vi "House.vi"() -> ()   [LabVIEW 2011]
panel:
  in  "WindowsMediaPlayer 2":refnum<k7>(container)
  out "Boolean 54":bool
  out "Boolean 53":bool
  out "Boolean 52":bool
  in  "stop 3":bool
  out "Boolean 51":bool
  out "LivingRoom2 Temprature":i32(slide) scale=1.0..60.0
  out "Bedroom2 Temprature":i32(slide) scale=1.0..60.0
  out "MasterRoom Temprature":i32(slide) scale=1.0..60.0
  out "DiningRoom Temprature":i32(slide) scale=1.0..60.0
  out "LivingRoom Temprature":i32(slide) scale=1.0..60.0
  in  "WindowsMediaPlayer":refnum<k7>(container)
  in  "stop 2":bool
  out "Bedroom Temprature":i32(slide) scale=1.0..60.0
  out "Boolean 50":bool
  out "Boolean 49":bool
  out "Boolean 48":bool
  out "Boolean 47":bool
  out "Boolean 46":bool
  out "Boolean 45":bool
  out "Slide 25":u8(slide)
  out "Slide 27":u8(slide)
  out "Horizontal Progress Bar":u8(slide) scale=0.0..100.0
  out "Horizontal Progress Bar 2":u8(slide)
  out "Boolean 44":bool
  out "Boolean 43":bool
  out "Boolean 42":bool
  out "Boolean 41":bool
  out "Boolean 40":bool
  out "Boolean 39":bool
  out "Boolean 38":bool
  out "Slide 24":u8(slide)
  out "Slide 23":u8(slide) scale=0.0..100.0
  out "Slide 22":u8(slide) scale=0.0..100.0
  out "Slide 21":u8(slide)
  out "Slide 20":u8(slide)
  out "Slide 19":u8(slide) scale=0.0..100.0
  out "Slide 18":u8(slide)
  out "Slide 17":u8(slide) scale=0.0..100.0
  out "Slide 16":u8(slide) scale=0.0..100.0
  out "Slide 15":u8(slide)
  out "Slide 14":u8(slide) scale=0.0..100.0
  out "Slide 13":u8(slide)
  out "Slide 12":u8(slide) scale=0.0..100.0
  out "Slide 11":u8(slide)
  out "Boolean 37":bool
  out "Boolean 36":bool
  out "Boolean 35":bool
  out "Boolean 34":bool
  out "Boolean 33":bool
  out "Boolean 32":bool
  out "Boolean 31":bool
  out "Boolean 30":bool
  out "Boolean 29":bool
  out "Boolean 28":bool
  out "Boolean 27":bool
  out "Slide 10":u8(slide) scale=0.0..100.0
  out "Slide 9":u8(slide)
  out "Slide 8":u8(slide)
  out "Slide 7":u8(slide) scale=0.0..100.0
  out "Slide 6":u8(slide)
  out "Slide 5":u8(slide) scale=0.0..100.0
  out "Slide 4":u8(slide) scale=0.0..100.0
  out "Slide 3":u8(slide)
  out "Slide 2":u8(slide)
  out "Slide":u8(slide) scale=0.0..100.0
  out "Boolean 26":bool
  out "Boolean 25":bool
  out "Boolean 24":bool
  out "Boolean 23":bool
  out "Boolean 22":bool
  out "Boolean 21":bool
  out "Boolean 20":bool
  out "Boolean 19":bool
  out "Boolean 18":bool
  out "Boolean 17":bool
  out "Boolean 16":bool
  out "Boolean 15":bool
  out "Boolean 14":bool
  out "Boolean 13":bool
  out "Boolean 12":bool
  out "Boolean 11":bool
  out "Boolean 10":bool
  out "Boolean 9":bool
  out "Boolean 8":bool
  out "Boolean 7":bool
  out "Boolean 6":bool
  out "Boolean 5":bool
  out "Boolean 4":bool
  out "Boolean 3":bool
  out "Boolean 2":bool
  out "Boolean":bool
  in  "stop":bool
  # "Ground Floor"
  # "First Floor"
  # "Ground Floor"
  # "First Floor"
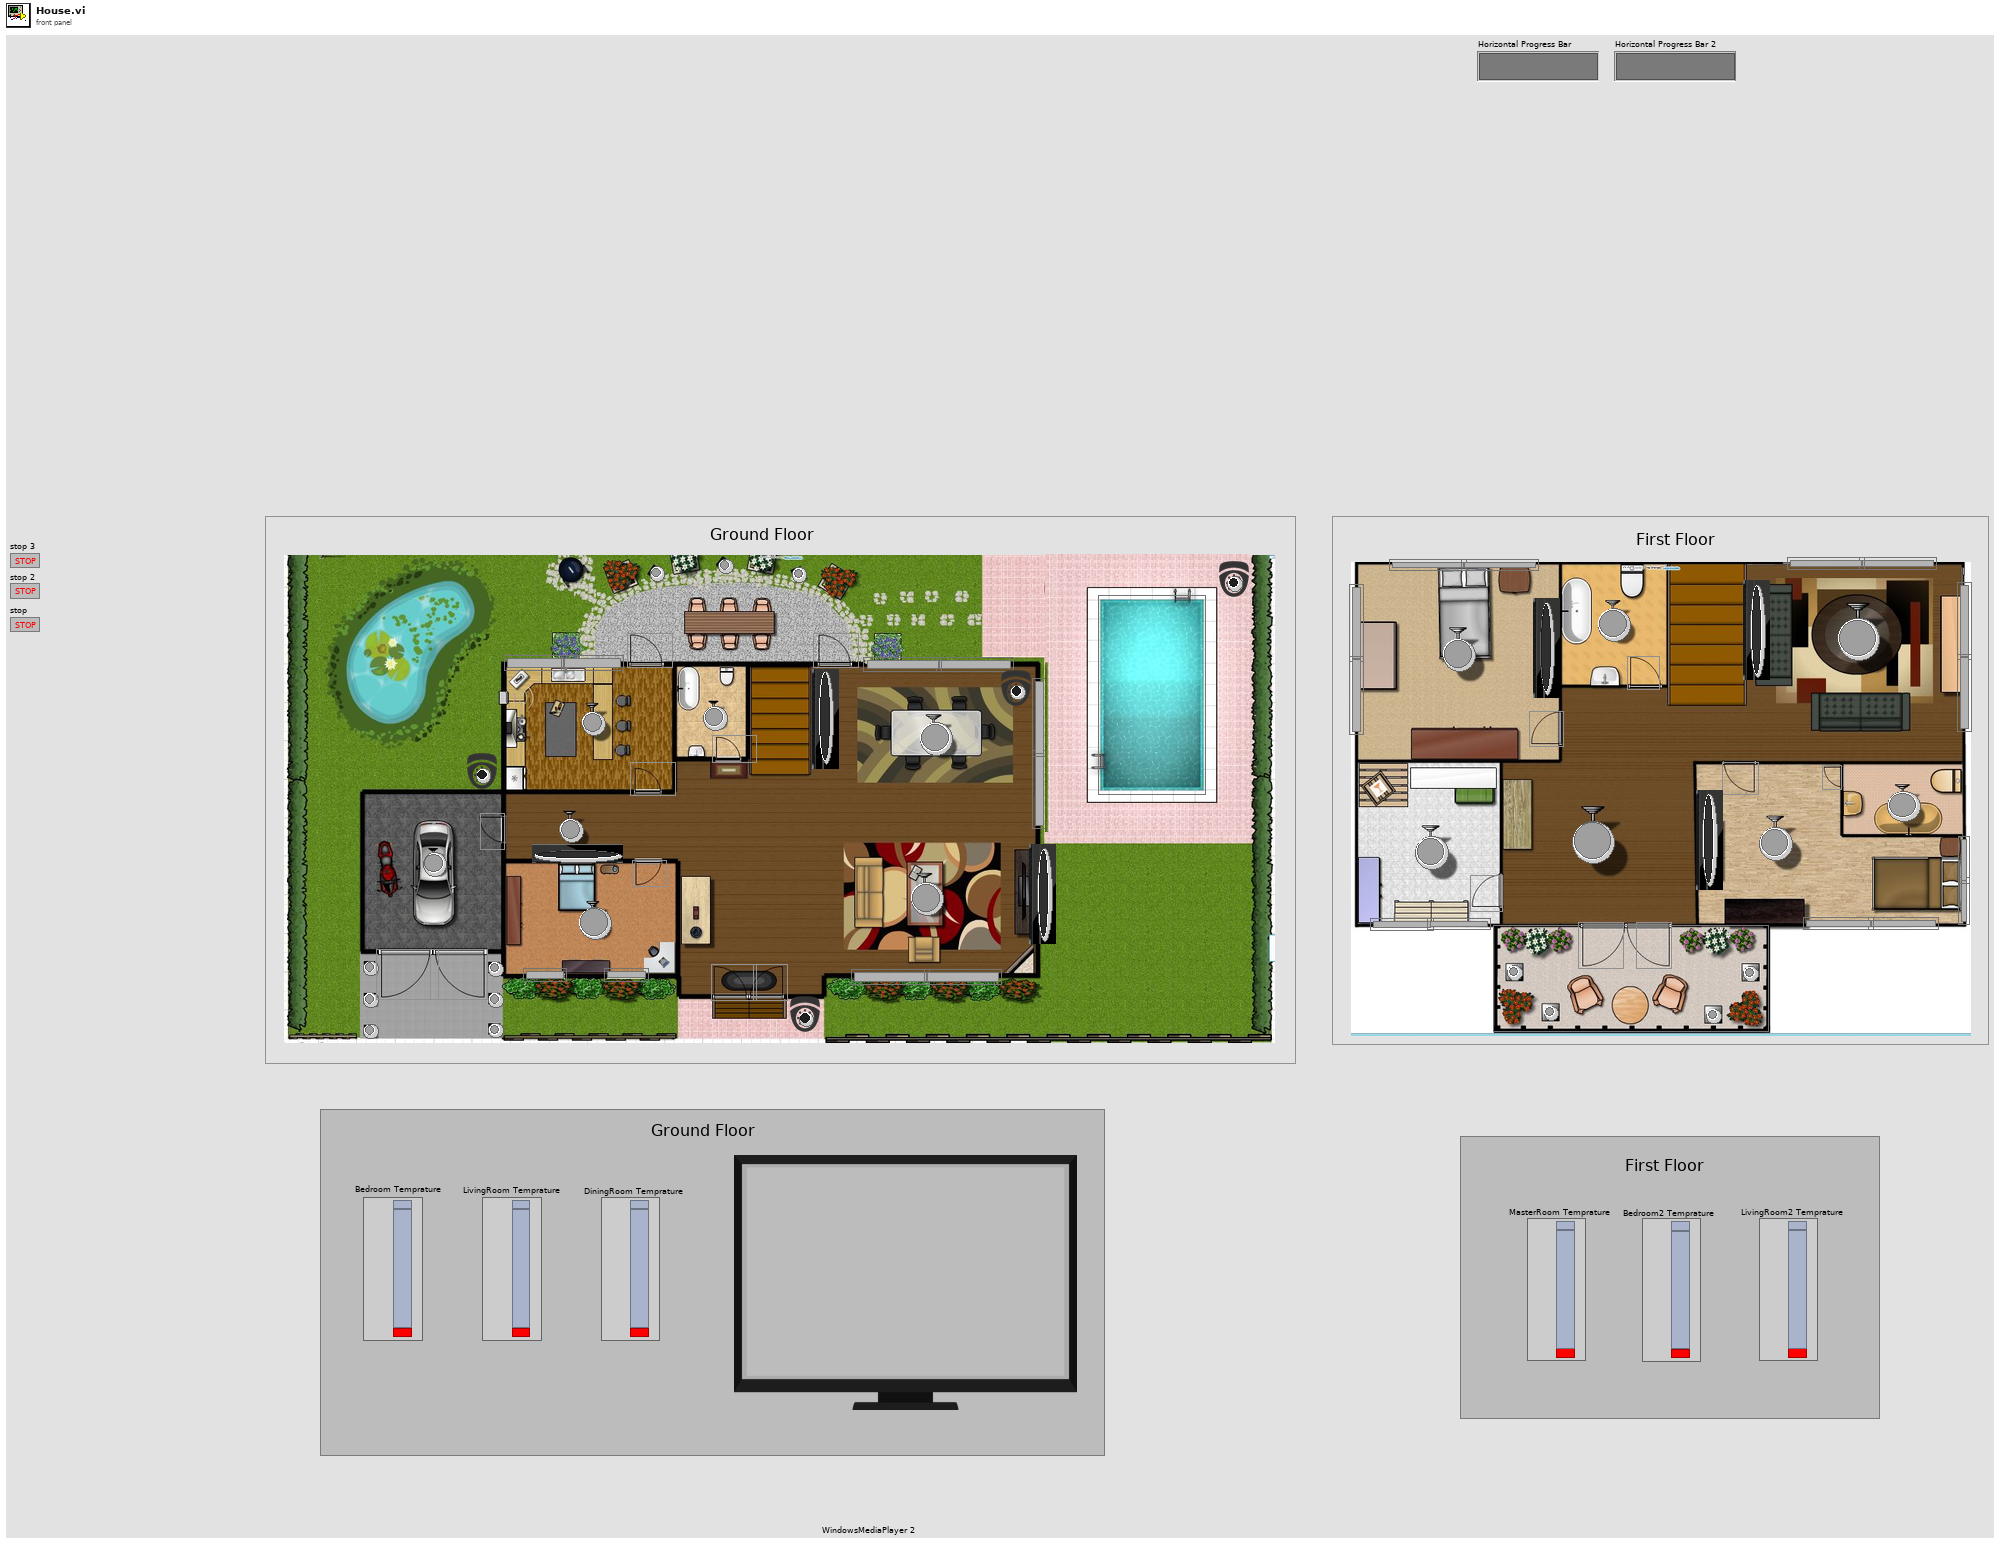
[diagram p1: front panel]
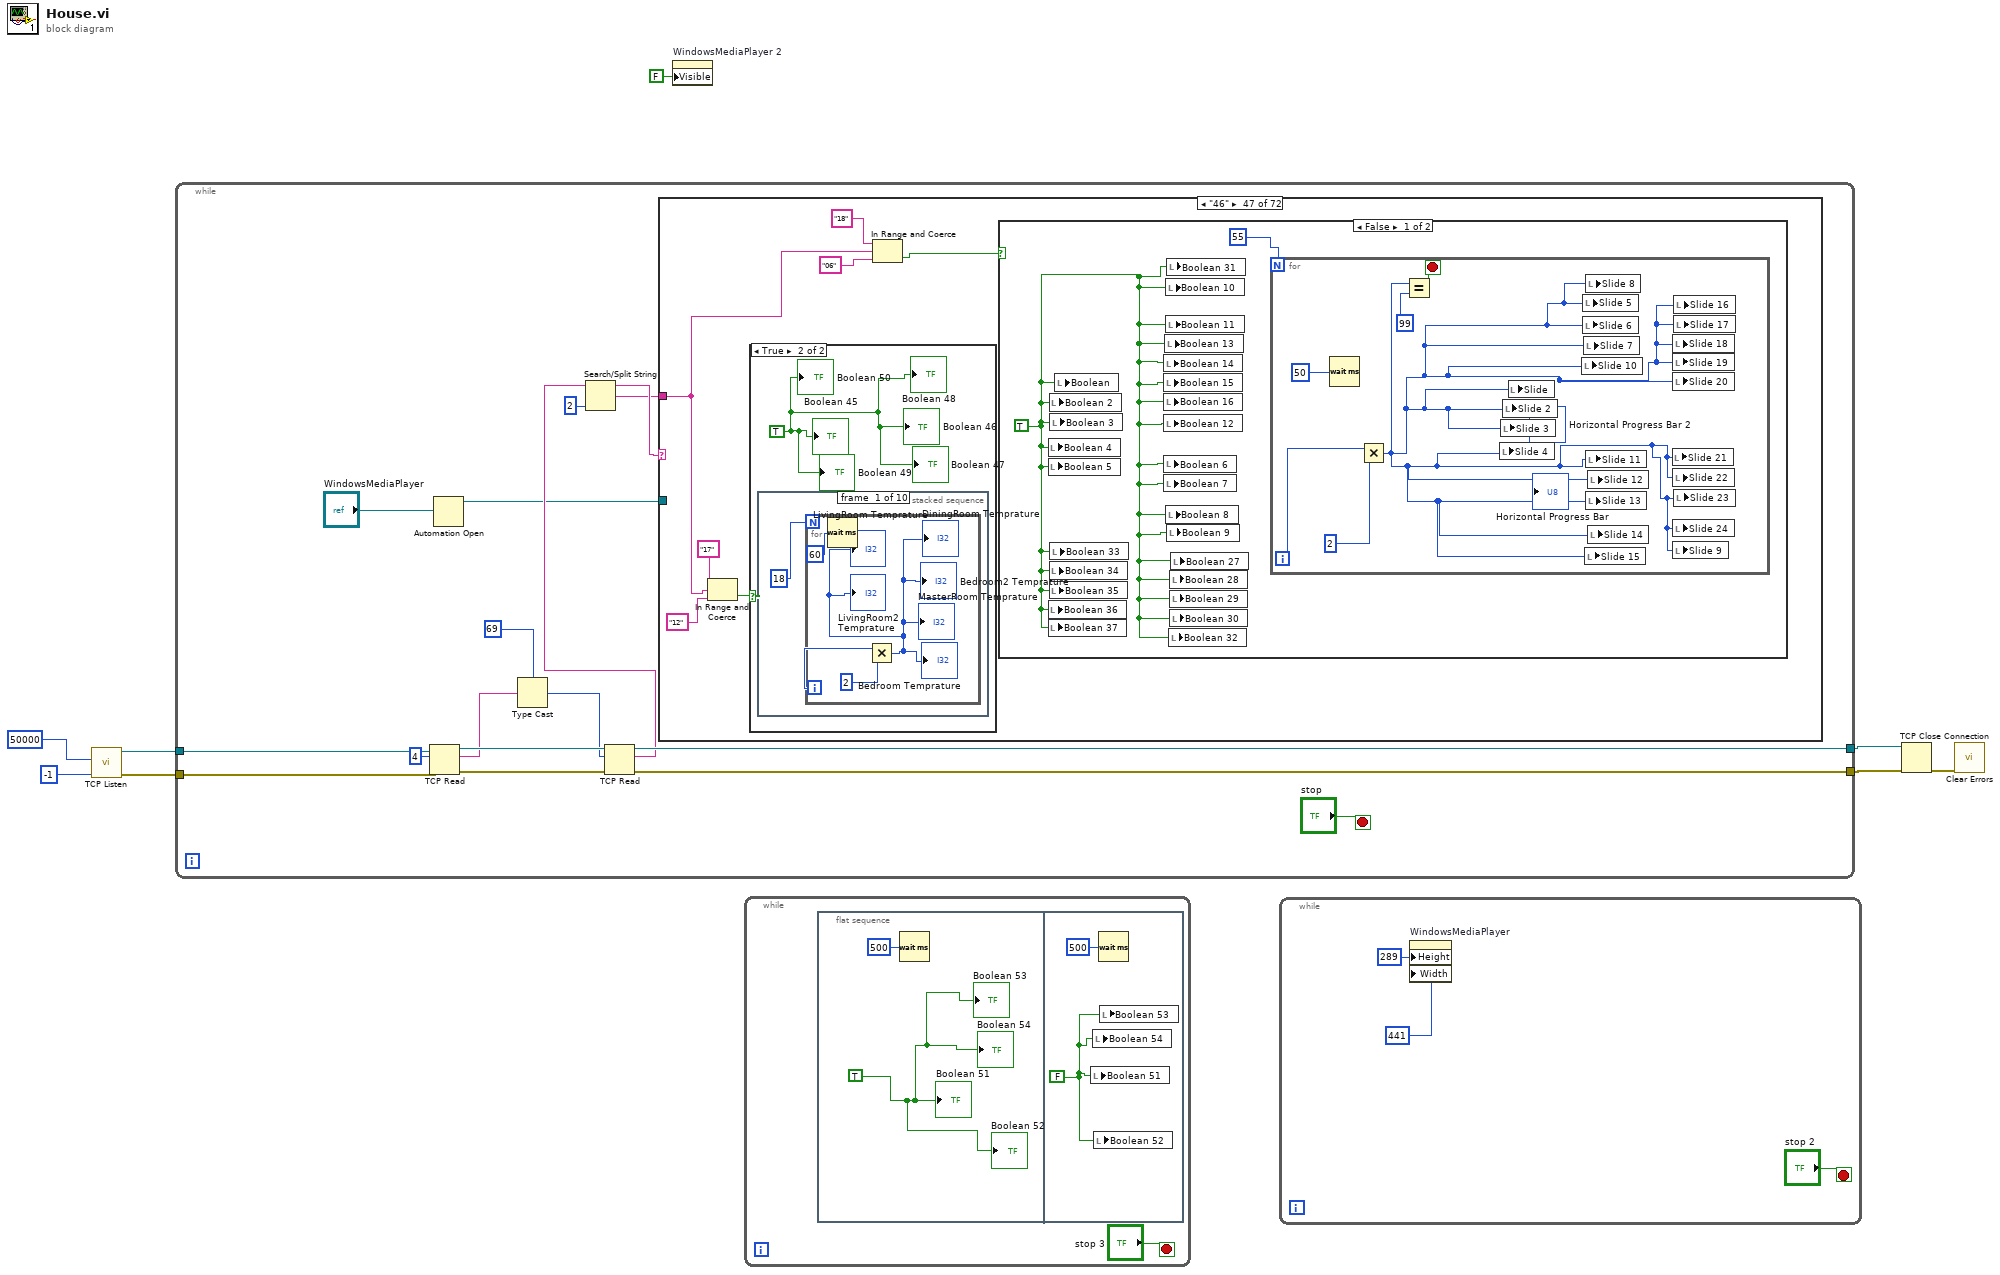
[diagram p0: block diagram]
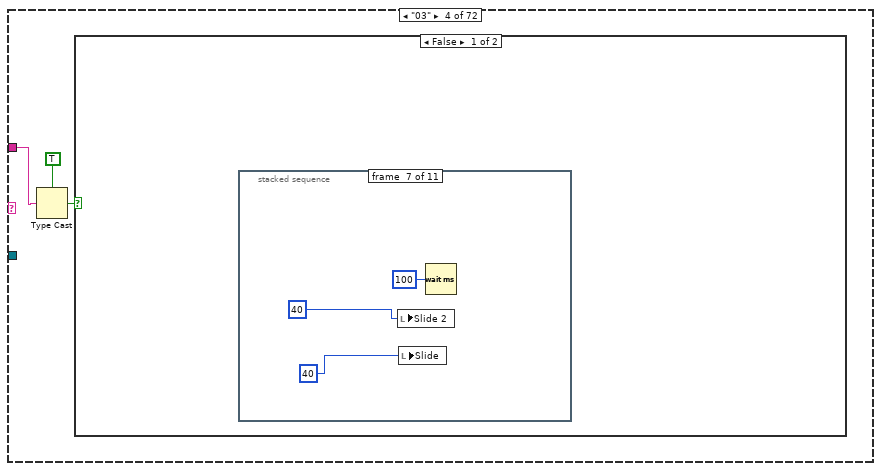
[diagram p5: hidden frame]
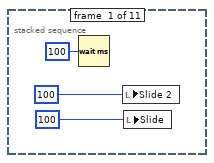
[diagram p6: hidden frame]
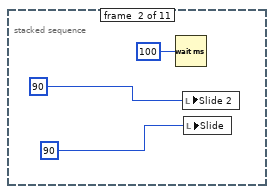
[diagram p7: hidden frame]
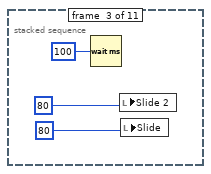
[diagram p8: hidden frame]
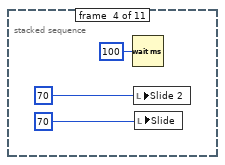
[diagram p9: hidden frame]
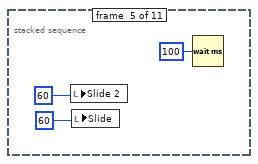
[diagram p10: hidden frame]
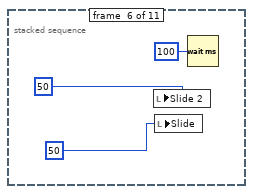
[diagram p11: hidden frame]
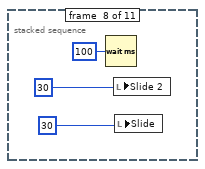
[diagram p12: hidden frame]
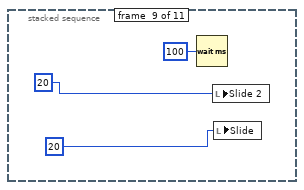
[diagram p13: hidden frame]
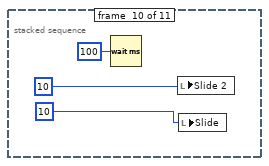
[diagram p14: hidden frame]
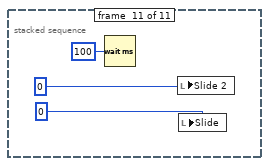
[diagram p15: hidden frame]
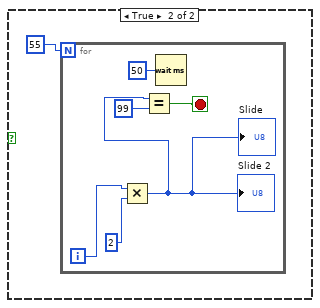
[diagram p16: hidden frame]
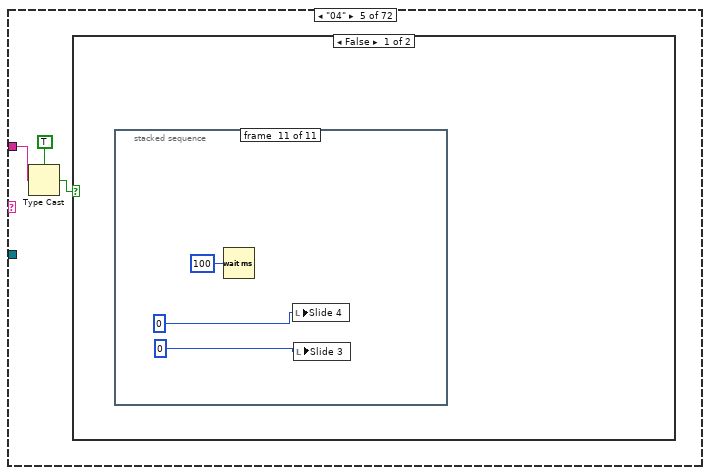
[diagram p17: hidden frame]
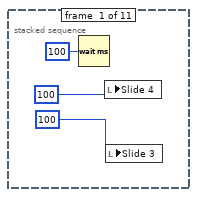
[diagram p18: hidden frame]
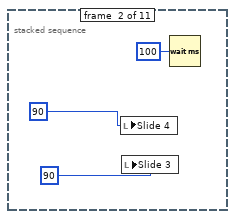
[diagram p19: hidden frame]
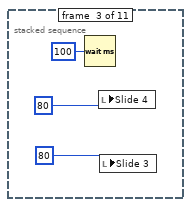
[diagram p20: hidden frame]
diagram:
  n1 = call <vilib>:"TCP Listen.vi"("timeout ms (wait forever: -1)"=-1, "port"=u16 50000) -> ("error out"=w6:errorcluster, "connection ID"=w8:refnum<k5>)  [unwired: 5 in, 3 out]
  n2 = while {
    tunnel: w8 -> [w25]
    tunnel: [w23] -> w7
    tunnel: w6 -> [w22]
    tunnel: [w9] -> w5
    stop <- "stop" stop-if-true
    n3 = TCP Read(connection ID=w25, bytes to read=4, error in (no error)=w22) -> (connection ID out=w24:refnum<k5>, data out=w19:string, error out=w21:errorcluster)  [unwired: 2 in]
    n4 = Automation Open(Automation Refnum="WindowsMediaPlayer") -> (Automation Refnum=w10:refnum<k7>)  [unwired: 3 in, 1 out]
    n5 = Type Cast(type=69, x=w19) -> (*(type *) &x=w18:i32)
    n6 = TCP Read(connection ID=w24, bytes to read=w18, error in (no error)=w21) -> (connection ID out=w23:refnum<k5>, data out=w15:string, error out=w9:errorcluster)  [unwired: 2 in]
    n7 = Search/Split String(string=w15, offset (0)=2) -> (substring before match=w13:string, match + rest of string=w12:string)  [unwired: 1 in, 1 out]
    n8 = case shown="\"46\"" w13 {
      tunnel: w12 -> [_ _ _ w27 w69 w112 w155 w199 w230 w263 w266 w269 w272 w275 w278 w281 w284 w298 w300 w303 w306 w309 w312 w315 w318 w321 w323 w355 w387 w420 w451 w483 w516 w519 w522 w525 w528 w531 w534 w537 w540 w543 w546 w549 w552 w555 w559 _ _ _ _ _ w635 w640 _ _ _ _ w654 w686 w719 w721 w723 w725 w727 w729 w731 w734 w737 w740 w743 w746]
      tunnel: w10 -> [_ _ _ _ _ _ _ _ _ _ _ _ _ _ _ _ _ _ _ _ _ _ _ _ _ _ _ _ _ _ _ _ _ _ _ _ _ _ _ _ _ _ _ _ _ _ _ w623 w626 w628 w630 w632 w638 w642 w644 w646 w648 w651 _ _ _ _ _ _ _ _ _ _ _ _ _ _]
      frame "False", Default {
      }
      frame "01" {
      }
      frame "02" {
      }
      frame "03" {
        n9 = Type Cast(type=TRUE, x=w27) -> (*(type *) &x=w28:bool)
        n10 = case shown="False" w28 {
          frame False {
            n11 = stacked-sequence {
              frame #0 {
                n12 = Wait (ms)(milliseconds to wait=u32 100) -> ()  [unwired: 1 out]
                n13 = local write "Slide 2"(u8 100 ("Horizontal Progress Bar 2")) -> ()
                n14 = local write "Slide"(u8 100 ("Horizontal Progress Bar")) -> ()
              }
              frame #1 {
                n15 = Wait (ms)(milliseconds to wait=u32 100) -> ()  [unwired: 1 out]
                n16 = local write "Slide 2"(u8 90 ("Horizontal Progress Bar 2")) -> ()
                n17 = local write "Slide"(u8 90 ("Horizontal Progress Bar")) -> ()
              }
              frame #2 {
                n18 = Wait (ms)(milliseconds to wait=u32 100) -> ()  [unwired: 1 out]
                n19 = local write "Slide 2"(u8 80 ("Horizontal Progress Bar 2")) -> ()
                n20 = local write "Slide"(u8 80 ("Horizontal Progress Bar")) -> ()
              }
              frame #3 {
                n21 = Wait (ms)(milliseconds to wait=u32 100) -> ()  [unwired: 1 out]
                n22 = local write "Slide 2"(u8 70 ("Horizontal Progress Bar 2")) -> ()
                n23 = local write "Slide"(u8 70 ("Horizontal Progress Bar")) -> ()
              }
              frame #4 {
                n24 = local write "Slide 2"(u8 60 ("Horizontal Progress Bar 2")) -> ()
                n25 = local write "Slide"(u8 60 ("Horizontal Progress Bar")) -> ()
                n26 = Wait (ms)(milliseconds to wait=u32 100) -> ()  [unwired: 1 out]
              }
              frame #5 {
                n27 = local write "Slide 2"(u8 50 ("Horizontal Progress Bar 2")) -> ()
                n28 = local write "Slide"(u8 50 ("Horizontal Progress Bar")) -> ()
                n29 = Wait (ms)(milliseconds to wait=u32 100) -> ()  [unwired: 1 out]
              }
              frame #6 {
                n30 = local write "Slide 2"(u8 40 ("Horizontal Progress Bar 2")) -> ()
                n31 = local write "Slide"(u8 40 ("Horizontal Progress Bar")) -> ()
                n32 = Wait (ms)(milliseconds to wait=u32 100) -> ()  [unwired: 1 out]
              }
              frame #7 {
                n33 = Wait (ms)(milliseconds to wait=u32 100) -> ()  [unwired: 1 out]
                n34 = local write "Slide 2"(u8 30 ("Horizontal Progress Bar 2")) -> ()
                n35 = local write "Slide"(u8 30 ("Horizontal Progress Bar")) -> ()
              }
              frame #8 {
                n36 = Wait (ms)(milliseconds to wait=u32 100) -> ()  [unwired: 1 out]
                n37 = local write "Slide 2"(u8 20 ("Horizontal Progress Bar 2")) -> ()
                n38 = local write "Slide"(u8 20 ("Horizontal Progress Bar")) -> ()
              }
              frame #9 {
                n39 = Wait (ms)(milliseconds to wait=u32 100) -> ()  [unwired: 1 out]
                n40 = local write "Slide 2"(u8 10 ("Horizontal Progress Bar 2")) -> ()
                n41 = local write "Slide"(u8 10 ("Horizontal Progress Bar")) -> ()
              }
              frame #10 {
                n42 = Wait (ms)(milliseconds to wait=u32 100) -> ()  [unwired: 1 out]
                n43 = local write "Slide 2"(u8 0 ("Horizontal Progress Bar 2")) -> ()
                n44 = local write "Slide"(u8 0 ("Horizontal Progress Bar")) -> ()
              }
            }
          }
          frame True {
            n45 = for {
              N: 55 -> [_]
              i -> [w68]
              stop <- w64 stop-if-true
              n46 = Multiply(x=w68, y=2) -> (x*y=w66:i32)
              "Slide" <- w66
              "Slide 2" <- w66
              n47 = Equal?(x=w66, y=99) -> (x = y?=w64:bool)
              n48 = Wait (ms)(milliseconds to wait=u32 50) -> ()  [unwired: 1 out]
            }
          }
        }
      }
      frame "04" {
        n49 = Type Cast(type=TRUE, x=w69) -> (*(type *) &x=w70:bool)
        n50 = case shown="False" w70 {
          frame False {
            n51 = stacked-sequence {
              frame #0 {
                n52 = Wait (ms)(milliseconds to wait=u32 100) -> ()  [unwired: 1 out]
                n53 = local write "Slide 4"(u8 100 ("Horizontal Progress Bar 2")) -> ()
                n54 = local write "Slide 3"(u8 100 ("Horizontal Progress Bar")) -> ()
              }
              frame #1 {
                n55 = local write "Slide 4"(u8 90 ("Horizontal Progress Bar 2")) -> ()
                n56 = local write "Slide 3"(u8 90 ("Horizontal Progress Bar")) -> ()
                n57 = Wait (ms)(milliseconds to wait=u32 100) -> ()  [unwired: 1 out]
              }
              frame #2 {
                n58 = Wait (ms)(milliseconds to wait=u32 100) -> ()  [unwired: 1 out]
                n59 = local write "Slide 4"(u8 80 ("Horizontal Progress Bar 2")) -> ()
                n60 = local write "Slide 3"(u8 80 ("Horizontal Progress Bar")) -> ()
              }
              frame #3 {
                n61 = local write "Slide 4"(u8 70 ("Horizontal Progress Bar 2")) -> ()
                n62 = local write "Slide 3"(u8 70 ("Horizontal Progress Bar")) -> ()
                n63 = Wait (ms)(milliseconds to wait=u32 100) -> ()  [unwired: 1 out]
              }
              frame #4 {
                n64 = local write "Slide 4"(u8 60 ("Horizontal Progress Bar 2")) -> ()
                n65 = local write "Slide 3"(u8 60 ("Horizontal Progress Bar")) -> ()
                n66 = Wait (ms)(milliseconds to wait=u32 100) -> ()  [unwired: 1 out]
              }
              frame #5 {
                n67 = Wait (ms)(milliseconds to wait=u32 100) -> ()  [unwired: 1 out]
                n68 = local write "Slide 4"(u8 50 ("Horizontal Progress Bar 2")) -> ()
                n69 = local write "Slide 3"(u8 50 ("Horizontal Progress Bar")) -> ()
              }
              frame #6 {
                n70 = local write "Slide 4"(u8 40 ("Horizontal Progress Bar 2")) -> ()
                n71 = local write "Slide 3"(u8 40 ("Horizontal Progress Bar")) -> ()
                n72 = Wait (ms)(milliseconds to wait=u32 100) -> ()  [unwired: 1 out]
              }
              frame #7 {
                n73 = Wait (ms)(milliseconds to wait=u32 100) -> ()  [unwired: 1 out]
                n74 = local write "Slide 4"(u8 30 ("Horizontal Progress Bar 2")) -> ()
                n75 = local write "Slide 3"(u8 30 ("Horizontal Progress Bar")) -> ()
              }
              frame #8 {
                n76 = Wait (ms)(milliseconds to wait=u32 100) -> ()  [unwired: 1 out]
                n77 = local write "Slide 4"(u8 20 ("Horizontal Progress Bar 2")) -> ()
                n78 = local write "Slide 3"(u8 20 ("Horizontal Progress Bar")) -> ()
              }
              frame #9 {
                n79 = Wait (ms)(milliseconds to wait=u32 100) -> ()  [unwired: 1 out]
                n80 = local write "Slide 4"(u8 10 ("Horizontal Progress Bar 2")) -> ()
                n81 = local write "Slide 3"(u8 10 ("Horizontal Progress Bar")) -> ()
              }
              frame #10 {
                n82 = Wait (ms)(milliseconds to wait=u32 100) -> ()  [unwired: 1 out]
                n83 = local write "Slide 4"(u8 0 ("Horizontal Progress Bar 2")) -> ()
                n84 = local write "Slide 3"(u8 0 ("Horizontal Progress Bar")) -> ()
              }
            }
          }
          frame True {
            n85 = for {
              N: 55 -> [_]
              i -> [w111]
              stop <- w108 stop-if-true
              n86 = Multiply(x=w111, y=2) -> (x*y=w106:i32)
              "Slide 3" <- w106
              "Slide 4" <- w106
              n87 = Equal?(x=w106, y=99) -> (x = y?=w108:bool)
              n88 = Wait (ms)(milliseconds to wait=u32 50) -> ()  [unwired: 1 out]
            }
          }
        }
      }
      frame "05" {
        n89 = Type Cast(type=TRUE, x=w112) -> (*(type *) &x=w113:bool)
        n90 = case shown="False" w113 {
          frame False {
            n91 = stacked-sequence {
              frame #0 {
                n92 = Wait (ms)(milliseconds to wait=u32 100) -> ()  [unwired: 1 out]
                n93 = local write "Slide 6"(u8 100 ("Horizontal Progress Bar 2")) -> ()
                n94 = local write "Slide 5"(u8 100 ("Horizontal Progress Bar")) -> ()
              }
              frame #1 {
                n95 = local write "Slide 6"(u8 90 ("Horizontal Progress Bar 2")) -> ()
                n96 = local write "Slide 5"(u8 90 ("Horizontal Progress Bar")) -> ()
                n97 = Wait (ms)(milliseconds to wait=u32 100) -> ()  [unwired: 1 out]
              }
              frame #2 {
                n98 = Wait (ms)(milliseconds to wait=u32 100) -> ()  [unwired: 1 out]
                n99 = local write "Slide 6"(u8 80 ("Horizontal Progress Bar 2")) -> ()
                n100 = local write "Slide 5"(u8 80 ("Horizontal Progress Bar")) -> ()
              }
              frame #3 {
                n101 = local write "Slide 6"(u8 70 ("Horizontal Progress Bar 2")) -> ()
                n102 = local write "Slide 5"(u8 70 ("Horizontal Progress Bar")) -> ()
                n103 = Wait (ms)(milliseconds to wait=u32 100) -> ()  [unwired: 1 out]
              }
              frame #4 {
                n104 = local write "Slide 6"(u8 60 ("Horizontal Progress Bar 2")) -> ()
                n105 = local write "Slide 5"(u8 60 ("Horizontal Progress Bar")) -> ()
                n106 = Wait (ms)(milliseconds to wait=u32 100) -> ()  [unwired: 1 out]
              }
              frame #5 {
                n107 = local write "Slide 6"(u8 50 ("Horizontal Progress Bar 2")) -> ()
                n108 = local write "Slide 5"(u8 50 ("Horizontal Progress Bar")) -> ()
                n109 = Wait (ms)(milliseconds to wait=u32 100) -> ()  [unwired: 1 out]
              }
              frame #6 {
                n110 = local write "Slide 6"(u8 40 ("Horizontal Progress Bar 2")) -> ()
                n111 = local write "Slide 5"(u8 40 ("Horizontal Progress Bar")) -> ()
                n112 = Wait (ms)(milliseconds to wait=u32 100) -> ()  [unwired: 1 out]
              }
              frame #7 {
                n113 = Wait (ms)(milliseconds to wait=u32 100) -> ()  [unwired: 1 out]
                n114 = local write "Slide 6"(u8 30 ("Horizontal Progress Bar 2")) -> ()
                n115 = local write "Slide 5"(u8 30 ("Horizontal Progress Bar")) -> ()
              }
              frame #8 {
                n116 = local write "Slide 6"(u8 20 ("Horizontal Progress Bar 2")) -> ()
                n117 = local write "Slide 5"(u8 20 ("Horizontal Progress Bar")) -> ()
                n118 = Wait (ms)(milliseconds to wait=u32 100) -> ()  [unwired: 1 out]
              }
              frame #9 {
                n119 = Wait (ms)(milliseconds to wait=u32 100) -> ()  [unwired: 1 out]
                n120 = local write "Slide 6"(u8 10 ("Horizontal Progress Bar 2")) -> ()
                n121 = local write "Slide 5"(u8 10 ("Horizontal Progress Bar")) -> ()
              }
              frame #10 {
                n122 = Wait (ms)(milliseconds to wait=u32 100) -> ()  [unwired: 1 out]
                n123 = local write "Slide 6"(u8 0 ("Horizontal Progress Bar 2")) -> ()
                n124 = local write "Slide 5"(u8 0 ("Horizontal Progress Bar")) -> ()
              }
            }
          }
          frame True {
            n125 = for {
              N: 55 -> [_]
              i -> [w154]
              stop <- w151 stop-if-true
              n126 = Multiply(x=w154, y=2) -> (x*y=w149:i32)
              "Slide 5" <- w149
              "Slide 6" <- w149
              n127 = Equal?(x=w149, y=99) -> (x = y?=w151:bool)
              n128 = Wait (ms)(milliseconds to wait=u32 50) -> ()  [unwired: 1 out]
            }
          }
        }
      }
      frame "06" {
        n129 = Type Cast(type=TRUE, x=w155) -> (*(type *) &x=w156:bool)
        n130 = case shown="False" w156 {
          frame False {
            n131 = stacked-sequence {
              frame #0 {
                n132 = Wait (ms)(milliseconds to wait=u32 100) -> ()  [unwired: 1 out]
                n133 = local write "Slide 8"(u8 100 ("Horizontal Progress Bar")) -> ()
                n134 = local write "Slide 7"(u8 100 ("Horizontal Progress Bar 2")) -> ()
              }
              frame #1 {
                n135 = Wait (ms)(milliseconds to wait=u32 100) -> ()  [unwired: 1 out]
                n136 = local write "Slide 8"(u8 90 ("Horizontal Progress Bar")) -> ()
                n137 = local write "Slide 7"(u8 90 ("Horizontal Progress Bar 2")) -> ()
              }
              frame #2 {
                n138 = Wait (ms)(milliseconds to wait=u32 100) -> ()  [unwired: 1 out]
                n139 = local write "Slide 8"(u8 80 ("Horizontal Progress Bar")) -> ()
                n140 = local write "Slide 7"(u8 80 ("Horizontal Progress Bar 2")) -> ()
              }
              frame #3 {
                n141 = Wait (ms)(milliseconds to wait=u32 100) -> ()  [unwired: 1 out]
                n142 = local write "Slide 8"(u8 70 ("Horizontal Progress Bar")) -> ()
                n143 = local write "Slide 7"(u8 70 ("Horizontal Progress Bar 2")) -> ()
              }
              frame #4 {
                n144 = local write "Slide 8"(u8 60 ("Horizontal Progress Bar")) -> ()
                n145 = Wait (ms)(milliseconds to wait=u32 100) -> ()  [unwired: 1 out]
                n146 = local write "Slide 7"(u8 60 ("Horizontal Progress Bar 2")) -> ()
              }
              frame #5 {
                n147 = Wait (ms)(milliseconds to wait=u32 100) -> ()  [unwired: 1 out]
                n148 = local write "Slide 8"(u8 50 ("Horizontal Progress Bar")) -> ()
                n149 = local write "Slide 7"(u8 50 ("Horizontal Progress Bar 2")) -> ()
              }
              frame #6 {
                n150 = Wait (ms)(milliseconds to wait=u32 100) -> ()  [unwired: 1 out]
                n151 = local write "Slide 8"(u8 40 ("Horizontal Progress Bar")) -> ()
                n152 = local write "Slide 7"(u8 40 ("Horizontal Progress Bar 2")) -> ()
              }
              frame #7 {
                n153 = Wait (ms)(milliseconds to wait=u32 100) -> ()  [unwired: 1 out]
                n154 = local write "Slide 8"(u8 30 ("Horizontal Progress Bar")) -> ()
                n155 = local write "Slide 7"(u8 30 ("Horizontal Progress Bar 2")) -> ()
              }
              frame #8 {
                n156 = local write "Slide 8"(u8 20 ("Horizontal Progress Bar")) -> ()
                n157 = Wait (ms)(milliseconds to wait=u32 100) -> ()  [unwired: 1 out]
                n158 = local write "Slide 7"(u8 20 ("Horizontal Progress Bar 2")) -> ()
              }
              frame #9 {
                n159 = Wait (ms)(milliseconds to wait=u32 100) -> ()  [unwired: 1 out]
                n160 = local write "Slide 8"(u8 10 ("Horizontal Progress Bar")) -> ()
                n161 = local write "Slide 7"(u8 10 ("Horizontal Progress Bar 2")) -> ()
              }
              frame #10 {
                n162 = Wait (ms)(milliseconds to wait=u32 100) -> ()  [unwired: 1 out]
                n163 = local write "Slide 8"(u8 0 ("Horizontal Progress Bar")) -> ()
                n164 = local write "Slide 7"(u8 0 ("Horizontal Progress Bar 2")) -> ()
              }
            }
          }
          frame True {
            n165 = for {
              N: 55 -> [_]
              i -> [w197]
              stop <- w194 stop-if-true
              n166 = Multiply(x=w197, y=2) -> (x*y=w192:i32)
              "Slide 7" <- w192
              "Slide 8" <- w192
              n167 = Equal?(x=w192, y=99) -> (x = y?=w194:bool)
              n168 = Wait (ms)(milliseconds to wait=u32 50) -> ()  [unwired: 1 out]
            }
          }
        }
      }
      frame "07" {
        n169 = Type Cast(type=TRUE, x=w199) -> (*(type *) &x=w198:bool)
        n170 = case shown="False" w198 {
          frame False {
            n171 = stacked-sequence {
              frame #0 {
                n172 = Wait (ms)(milliseconds to wait=u32 100) -> ()  [unwired: 1 out]
                n173 = local write "Slide 9"(u8 100 ("Horizontal Progress Bar 2")) -> ()
              }
              frame #1 {
                n174 = local write "Slide 9"(u8 90 ("Horizontal Progress Bar 2")) -> ()
                n175 = Wait (ms)(milliseconds to wait=u32 100) -> ()  [unwired: 1 out]
              }
              frame #2 {
                n176 = Wait (ms)(milliseconds to wait=u32 100) -> ()  [unwired: 1 out]
                n177 = local write "Slide 9"(u8 80 ("Horizontal Progress Bar 2")) -> ()
              }
              frame #3 {
                n178 = local write "Slide 9"(u8 70 ("Horizontal Progress Bar 2")) -> ()
                n179 = Wait (ms)(milliseconds to wait=u32 100) -> ()  [unwired: 1 out]
              }
              frame #4 {
                n180 = local write "Slide 9"(u8 60 ("Horizontal Progress Bar 2")) -> ()
                n181 = Wait (ms)(milliseconds to wait=u32 100) -> ()  [unwired: 1 out]
              }
              frame #5 {
                n182 = local write "Slide 9"(u8 50 ("Horizontal Progress Bar 2")) -> ()
                n183 = Wait (ms)(milliseconds to wait=u32 100) -> ()  [unwired: 1 out]
              }
              frame #6 {
                n184 = local write "Slide 9"(u8 40 ("Horizontal Progress Bar 2")) -> ()
                n185 = Wait (ms)(milliseconds to wait=u32 100) -> ()  [unwired: 1 out]
              }
              frame #7 {
                n186 = Wait (ms)(milliseconds to wait=u32 100) -> ()  [unwired: 1 out]
                n187 = local write "Slide 9"(u8 30 ("Horizontal Progress Bar 2")) -> ()
              }
              frame #8 {
                n188 = local write "Slide 9"(u8 20 ("Horizontal Progress Bar 2")) -> ()
                n189 = Wait (ms)(milliseconds to wait=u32 100) -> ()  [unwired: 1 out]
              }
              frame #9 {
                n190 = Wait (ms)(milliseconds to wait=u32 100) -> ()  [unwired: 1 out]
                n191 = local write "Slide 9"(u8 10 ("Horizontal Progress Bar 2")) -> ()
              }
              frame #10 {
                n192 = Wait (ms)(milliseconds to wait=u32 100) -> ()  [unwired: 1 out]
                n193 = local write "Slide 9"(u8 0 ("Horizontal Progress Bar 2")) -> ()
              }
            }
          }
          frame True {
            n194 = for {
              N: 55 -> [_]
              i -> [w229]
              stop <- w226 stop-if-true
              n195 = Multiply(x=w229, y=2) -> (x*y=w224:i32)
              "Slide 9" <- w224
              n196 = Equal?(x=w224, y=99) -> (x = y?=w226:bool)
              n197 = Wait (ms)(milliseconds to wait=u32 50) -> ()  [unwired: 1 out]
            }
          }
        }
      }
      frame "08" {
        n198 = Type Cast(type=TRUE, x=w230) -> (*(type *) &x=w232:bool)
        n199 = case shown="False" w232 {
          frame False {
            n200 = stacked-sequence {
              frame #0 {
                n201 = Wait (ms)(milliseconds to wait=u32 100) -> ()  [unwired: 1 out]
                n202 = local write "Slide 10"(u8 100 ("Horizontal Progress Bar 2")) -> ()
              }
              frame #1 {
                n203 = local write "Slide 10"(u8 90 ("Horizontal Progress Bar 2")) -> ()
                n204 = Wait (ms)(milliseconds to wait=u32 100) -> ()  [unwired: 1 out]
              }
              frame #2 {
                n205 = local write "Slide 10"(u8 80 ("Horizontal Progress Bar 2")) -> ()
                n206 = Wait (ms)(milliseconds to wait=u32 100) -> ()  [unwired: 1 out]
              }
              frame #3 {
                n207 = local write "Slide 10"(u8 70 ("Horizontal Progress Bar 2")) -> ()
                n208 = Wait (ms)(milliseconds to wait=u32 100) -> ()  [unwired: 1 out]
              }
              frame #4 {
                n209 = local write "Slide 10"(u8 60 ("Horizontal Progress Bar 2")) -> ()
                n210 = Wait (ms)(milliseconds to wait=u32 100) -> ()  [unwired: 1 out]
              }
              frame #5 {
                n211 = local write "Slide 10"(u8 50 ("Horizontal Progress Bar 2")) -> ()
                n212 = Wait (ms)(milliseconds to wait=u32 100) -> ()  [unwired: 1 out]
              }
              frame #6 {
                n213 = local write "Slide 10"(u8 40 ("Horizontal Progress Bar 2")) -> ()
                n214 = Wait (ms)(milliseconds to wait=u32 100) -> ()  [unwired: 1 out]
              }
              frame #7 {
                n215 = local write "Slide 10"(u8 30 ("Horizontal Progress Bar 2")) -> ()
                n216 = Wait (ms)(milliseconds to wait=u32 100) -> ()  [unwired: 1 out]
              }
              frame #8 {
                n217 = local write "Slide 10"(u8 20 ("Horizontal Progress Bar 2")) -> ()
                n218 = Wait (ms)(milliseconds to wait=u32 100) -> ()  [unwired: 1 out]
              }
              frame #9 {
                n219 = local write "Slide 10"(u8 10 ("Horizontal Progress Bar 2")) -> ()
                n220 = Wait (ms)(milliseconds to wait=u32 100) -> ()  [unwired: 1 out]
              }
              frame #10 {
                n221 = Wait (ms)(milliseconds to wait=u32 100) -> ()  [unwired: 1 out]
                n222 = local write "Slide 10"(u8 0 ("Horizontal Progress Bar 2")) -> ()
              }
            }
          }
          frame True {
            n223 = for {
              N: 55 -> [_]
              i -> [w261]
              stop <- w258 stop-if-true
              n224 = Multiply(x=w261, y=2) -> (x*y=w256:i32)
              "Slide 10" <- w256
              n225 = Equal?(x=w256, y=99) -> (x = y?=w258:bool)
              n226 = Wait (ms)(milliseconds to wait=u32 50) -> ()  [unwired: 1 out]
            }
          }
        }
      }
      frame "09" {
        n227 = Type Cast(type=TRUE, x=w263) -> (*(type *) &x=→"Boolean 17" →"Boolean 18":bool)
      }
      frame "10" {
        n228 = Type Cast(type=TRUE, x=w266) -> (*(type *) &x=→"Boolean 22":bool)
      }
      frame "11" {
        n229 = Type Cast(type=TRUE, x=w269) -> (*(type *) &x=→"Boolean 21":bool)
      }
      frame "12" {
        n230 = Type Cast(type=TRUE, x=w272) -> (*(type *) &x=→"Boolean 26":bool)
      }
      frame "13" {
        n231 = Type Cast(type=TRUE, x=w275) -> (*(type *) &x=→"Boolean 19":bool)
      }
      frame "14" {
        n232 = Type Cast(type=TRUE, x=w278) -> (*(type *) &x=→"Boolean 20":bool)
      }
      frame "15" {
        n233 = Type Cast(type=TRUE, x=w281) -> (*(type *) &x=→"Boolean 23":bool)
      }
      frame "16" {
        n234 = Type Cast(type=TRUE, x=w284) -> (*(type *) &x=w283:bool)
        n235 = case shown="True" w283 {
          frame False {
            n236 = local write "Boolean 24"(FALSE ("Boolean 24")) -> ()
            n237 = local write "Boolean 25"(FALSE ("Boolean 24")) -> ()
            n238 = local read "WindowsMediaPlayer 2"() -> (w286:refnum<k7>)
            n239 = property class="IWMPPlayer4"(reference=w286) -> ("controls"=w287:refnum<k7>)  [unwired: 1 in, 2 out]
            n240 = invoke class="IWMPControls" method="play"(reference=w287) -> ()  [unwired: 2 in, 3 out]
          }
          frame True {
            n241 = Automation Open(Automation Refnum="WindowsMediaPlayer 2") -> (Automation Refnum=w292:refnum<k7>)  [unwired: 3 in, 1 out]
            n242 = property class="IWMPPlayer4"(reference=w292, "URL"="E:\\spcc.mp3") -> ()  [unwired: 1 in, 2 out]
            n243 = property class="IWMPPlayer4"(reference=w292) -> ("controls"=w291:refnum<k7>)  [unwired: 1 in, 2 out]
            n244 = invoke class="IWMPControls" method="play"(reference=w291) -> ()  [unwired: 2 in, 3 out]
            "Boolean 25" <- TRUE ("Boolean 24")
            "Boolean 24" <- TRUE ("Boolean 24")
          }
        }
      }
      frame "17" {
        n245 = Type Cast(type=TRUE, x=w298) -> (*(type *) &x=→"Boolean":bool)
      }
      frame "18" {
        n246 = Type Cast(type=TRUE, x=w300) -> (*(type *) &x=→"Boolean 2":bool)
      }
      frame "19" {
        n247 = Type Cast(type=TRUE, x=w303) -> (*(type *) &x=→"Boolean 3":bool)
      }
      frame "20" {
        n248 = Type Cast(type=TRUE, x=w306) -> (*(type *) &x=→"Boolean 4":bool)
      }
      frame "21" {
        n249 = Type Cast(type=TRUE, x=w309) -> (*(type *) &x=→"Boolean 5":bool)
      }
      frame "22" {
        n250 = Type Cast(type=TRUE, x=w312) -> (*(type *) &x=→"Boolean 6":bool)
      }
      frame "23" {
        n251 = Type Cast(type=TRUE, x=w315) -> (*(type *) &x=→"Boolean 7":bool)
      }
      frame "24" {
        n252 = Type Cast(type=TRUE, x=w318) -> (*(type *) &x=→"Boolean 8" →"Boolean 10" →"Boolean 11" →"Boolean 12" →"Boolean 13" →"Boolean 14":bool)
      }
      frame "25" {
        n253 = Type Cast(type=TRUE, x=w321) -> (*(type *) &x=→"Boolean 9" →"Boolean 16" →"Boolean 15":bool)
      }
      frame "26" {
        n254 = Type Cast(type=TRUE, x=w323) -> (*(type *) &x=w325:bool)
        n255 = case shown="False" w325 {
          frame False {
            n256 = stacked-sequence {
              frame #0 {
                w326 = u8 100 ("Horizontal Progress Bar 2")
                n257 = Wait (ms)(milliseconds to wait=u32 100) -> ()  [unwired: 1 out]
                n258 = local write "Slide 13"(w326) -> ()
                n259 = local write "Slide 14"(w326) -> ()
                n260 = local write "Slide 11"(w326) -> ()
                n261 = local write "Slide 12"(w326) -> ()
              }
              frame #1 {
                w328 = u8 90 ("Horizontal Progress Bar 2")
                n262 = Wait (ms)(milliseconds to wait=u32 100) -> ()  [unwired: 1 out]
                n263 = local write "Slide 13"(w328) -> ()
                n264 = local write "Slide 14"(w328) -> ()
                n265 = local write "Slide 11"(w328) -> ()
                n266 = local write "Slide 12"(w328) -> ()
              }
              frame #2 {
                w330 = u8 80 ("Horizontal Progress Bar 2")
                n267 = Wait (ms)(milliseconds to wait=u32 100) -> ()  [unwired: 1 out]
                n268 = local write "Slide 13"(w330) -> ()
                n269 = local write "Slide 14"(w330) -> ()
                n270 = local write "Slide 11"(w330) -> ()
                n271 = local write "Slide 12"(w330) -> ()
              }
              frame #3 {
                w332 = u8 70 ("Horizontal Progress Bar 2")
                n272 = Wait (ms)(milliseconds to wait=u32 100) -> ()  [unwired: 1 out]
                n273 = local write "Slide 13"(w332) -> ()
                n274 = local write "Slide 14"(w332) -> ()
                n275 = local write "Slide 11"(w332) -> ()
                n276 = local write "Slide 12"(w332) -> ()
              }
              frame #4 {
                w334 = u8 60 ("Horizontal Progress Bar 2")
                n277 = Wait (ms)(milliseconds to wait=u32 100) -> ()  [unwired: 1 out]
                n278 = local write "Slide 13"(w334) -> ()
                n279 = local write "Slide 14"(w334) -> ()
                n280 = local write "Slide 11"(w334) -> ()
                n281 = local write "Slide 12"(w334) -> ()
              }
              frame #5 {
                w336 = u8 50 ("Horizontal Progress Bar 2")
                n282 = Wait (ms)(milliseconds to wait=u32 100) -> ()  [unwired: 1 out]
                n283 = local write "Slide 13"(w336) -> ()
                n284 = local write "Slide 14"(w336) -> ()
                n285 = local write "Slide 11"(w336) -> ()
                n286 = local write "Slide 12"(w336) -> ()
              }
              frame #6 {
                w338 = u8 40 ("Horizontal Progress Bar 2")
                n287 = Wait (ms)(milliseconds to wait=u32 100) -> ()  [unwired: 1 out]
                n288 = local write "Slide 13"(w338) -> ()
                n289 = local write "Slide 14"(w338) -> ()
                n290 = local write "Slide 11"(w338) -> ()
                n291 = local write "Slide 12"(w338) -> ()
              }
              frame #7 {
                w340 = u8 30 ("Horizontal Progress Bar 2")
                n292 = Wait (ms)(milliseconds to wait=u32 100) -> ()  [unwired: 1 out]
                n293 = local write "Slide 13"(w340) -> ()
                n294 = local write "Slide 14"(w340) -> ()
                n295 = local write "Slide 11"(w340) -> ()
                n296 = local write "Slide 12"(w340) -> ()
              }
              frame #8 {
                w342 = u8 20 ("Horizontal Progress Bar 2")
                n297 = Wait (ms)(milliseconds to wait=u32 100) -> ()  [unwired: 1 out]
                n298 = local write "Slide 13"(w342) -> ()
                n299 = local write "Slide 14"(w342) -> ()
                n300 = local write "Slide 11"(w342) -> ()
                n301 = local write "Slide 12"(w342) -> ()
              }
              frame #9 {
                w344 = u8 10 ("Horizontal Progress Bar 2")
                n302 = Wait (ms)(milliseconds to wait=u32 100) -> ()  [unwired: 1 out]
                n303 = local write "Slide 13"(w344) -> ()
                n304 = local write "Slide 14"(w344) -> ()
                n305 = local write "Slide 11"(w344) -> ()
                n306 = local write "Slide 12"(w344) -> ()
              }
              frame #10 {
                w346 = u8 0 ("Horizontal Progress Bar 2")
                n307 = Wait (ms)(milliseconds to wait=u32 100) -> ()  [unwired: 1 out]
                n308 = local write "Slide 13"(w346) -> ()
                n309 = local write "Slide 14"(w346) -> ()
                n310 = local write "Slide 11"(w346) -> ()
                n311 = local write "Slide 12"(w346) -> ()
              }
            }
          }
          frame True {
            n312 = for {
              N: 55 -> [_]
              i -> [w354]
              stop <- w351 stop-if-true
              n313 = Multiply(x=w354, y=2) -> (x*y=w349:i32)
              "Slide 11" <- w349
              "Slide 12" <- w349
              "Slide 14" <- w349
              "Slide 13" <- w349
              n314 = Equal?(x=w349, y=99) -> (x = y?=w351:bool)
              n315 = Wait (ms)(milliseconds to wait=u32 50) -> ()  [unwired: 1 out]
            }
          }
        }
      }
      frame "27" {
        n316 = Type Cast(type=TRUE, x=w355) -> (*(type *) &x=w356:bool)
        n317 = case shown="False" w356 {
          frame False {
            n318 = stacked-sequence {
              frame #0 {
                w358 = u8 100 ("Horizontal Progress Bar 2")
                n319 = Wait (ms)(milliseconds to wait=u32 100) -> ()  [unwired: 1 out]
                n320 = local write "Slide 15"(w358) -> ()
                n321 = local write "Slide 16"(w358) -> ()
              }
              frame #1 {
                w360 = u8 90 ("Horizontal Progress Bar 2")
                n322 = local write "Slide 15"(w360) -> ()
                n323 = local write "Slide 16"(w360) -> ()
                n324 = Wait (ms)(milliseconds to wait=u32 100) -> ()  [unwired: 1 out]
              }
              frame #2 {
                w362 = u8 80 ("Horizontal Progress Bar 2")
                n325 = Wait (ms)(milliseconds to wait=u32 100) -> ()  [unwired: 1 out]
                n326 = local write "Slide 15"(w362) -> ()
                n327 = local write "Slide 16"(w362) -> ()
              }
              frame #3 {
                w364 = u8 70 ("Horizontal Progress Bar 2")
                n328 = Wait (ms)(milliseconds to wait=u32 100) -> ()  [unwired: 1 out]
                n329 = local write "Slide 15"(w364) -> ()
                n330 = local write "Slide 16"(w364) -> ()
              }
              frame #4 {
                w366 = u8 60 ("Horizontal Progress Bar 2")
                n331 = local write "Slide 15"(w366) -> ()
                n332 = local write "Slide 16"(w366) -> ()
                n333 = Wait (ms)(milliseconds to wait=u32 100) -> ()  [unwired: 1 out]
              }
              frame #5 {
                w368 = u8 50 ("Horizontal Progress Bar 2")
                n334 = Wait (ms)(milliseconds to wait=u32 100) -> ()  [unwired: 1 out]
                n335 = local write "Slide 15"(w368) -> ()
                n336 = local write "Slide 16"(w368) -> ()
              }
              frame #6 {
                w370 = u8 40 ("Horizontal Progress Bar 2")
                n337 = Wait (ms)(milliseconds to wait=u32 100) -> ()  [unwired: 1 out]
                n338 = local write "Slide 15"(w370) -> ()
                n339 = local write "Slide 16"(w370) -> ()
              }
              frame #7 {
                w372 = u8 30 ("Horizontal Progress Bar 2")
                n340 = Wait (ms)(milliseconds to wait=u32 100) -> ()  [unwired: 1 out]
                n341 = local write "Slide 15"(w372) -> ()
                n342 = local write "Slide 16"(w372) -> ()
              }
              frame #8 {
                w374 = u8 20 ("Horizontal Progress Bar 2")
                n343 = Wait (ms)(milliseconds to wait=u32 100) -> ()  [unwired: 1 out]
                n344 = local write "Slide 15"(w374) -> ()
                n345 = local write "Slide 16"(w374) -> ()
              }
              frame #9 {
                w376 = u8 10 ("Horizontal Progress Bar 2")
                n346 = Wait (ms)(milliseconds to wait=u32 100) -> ()  [unwired: 1 out]
                n347 = local write "Slide 15"(w376) -> ()
                n348 = local write "Slide 16"(w376) -> ()
              }
              frame #10 {
                w378 = u8 0 ("Horizontal Progress Bar 2")
                n349 = Wait (ms)(milliseconds to wait=u32 100) -> ()  [unwired: 1 out]
                n350 = local write "Slide 15"(w378) -> ()
                n351 = local write "Slide 16"(w378) -> ()
              }
            }
          }
          frame True {
            n352 = for {
              N: 55 -> [_]
              i -> [w386]
              stop <- w383 stop-if-true
              n353 = Multiply(x=w386, y=2) -> (x*y=w381:i32)
              "Slide 15" <- w381
              "Slide 16" <- w381
              n354 = Equal?(x=w381, y=99) -> (x = y?=w383:bool)
              n355 = Wait (ms)(milliseconds to wait=u32 50) -> ()  [unwired: 1 out]
            }
          }
        }
      }
      frame "28" {
        n356 = Type Cast(type=TRUE, x=w387) -> (*(type *) &x=w388:bool)
        n357 = case shown="False" w388 {
          frame False {
            n358 = stacked-sequence {
              frame #0 {
                w390 = u8 100 ("Horizontal Progress Bar 2")
                n359 = Wait (ms)(milliseconds to wait=u32 100) -> ()  [unwired: 1 out]
                n360 = local write "Slide 18"(w390) -> ()
                n361 = local write "Slide 17"(w390) -> ()
              }
              frame #1 {
                w392 = u8 90 ("Horizontal Progress Bar 2")
                n362 = Wait (ms)(milliseconds to wait=u32 100) -> ()  [unwired: 1 out]
                n363 = local write "Slide 18"(w392) -> ()
                n364 = local write "Slide 17"(w392) -> ()
              }
              frame #2 {
                w394 = u8 80 ("Horizontal Progress Bar 2")
                n365 = Wait (ms)(milliseconds to wait=u32 100) -> ()  [unwired: 1 out]
                n366 = local write "Slide 18"(w394) -> ()
                n367 = local write "Slide 17"(w394) -> ()
              }
              frame #3 {
                w396 = u8 70 ("Horizontal Progress Bar 2")
                n368 = Wait (ms)(milliseconds to wait=u32 100) -> ()  [unwired: 1 out]
                n369 = local write "Slide 18"(w396) -> ()
                n370 = local write "Slide 17"(w396) -> ()
              }
              frame #4 {
                w398 = u8 60 ("Horizontal Progress Bar 2")
                n371 = Wait (ms)(milliseconds to wait=u32 100) -> ()  [unwired: 1 out]
                n372 = local write "Slide 18"(w398) -> ()
                n373 = local write "Slide 17"(w398) -> ()
              }
              frame #5 {
                w400 = u8 50 ("Horizontal Progress Bar 2")
                n374 = Wait (ms)(milliseconds to wait=u32 100) -> ()  [unwired: 1 out]
                n375 = local write "Slide 18"(w400) -> ()
                n376 = local write "Slide 17"(w400) -> ()
              }
              frame #6 {
                w402 = u8 40 ("Horizontal Progress Bar 2")
                n377 = Wait (ms)(milliseconds to wait=u32 100) -> ()  [unwired: 1 out]
                n378 = local write "Slide 18"(w402) -> ()
                n379 = local write "Slide 17"(w402) -> ()
              }
              frame #7 {
                w404 = u8 30 ("Horizontal Progress Bar 2")
                n380 = Wait (ms)(milliseconds to wait=u32 100) -> ()  [unwired: 1 out]
                n381 = local write "Slide 18"(w404) -> ()
                n382 = local write "Slide 17"(w404) -> ()
              }
              frame #8 {
                w406 = u8 20 ("Horizontal Progress Bar 2")
                n383 = Wait (ms)(milliseconds to wait=u32 100) -> ()  [unwired: 1 out]
                n384 = local write "Slide 18"(w406) -> ()
                n385 = local write "Slide 17"(w406) -> ()
              }
              frame #9 {
                w408 = u8 10 ("Horizontal Progress Bar 2")
                n386 = Wait (ms)(milliseconds to wait=u32 100) -> ()  [unwired: 1 out]
                n387 = local write "Slide 18"(w408) -> ()
                n388 = local write "Slide 17"(w408) -> ()
              }
              frame #10 {
                w410 = u8 0 ("Horizontal Progress Bar 2")
                n389 = Wait (ms)(milliseconds to wait=u32 100) -> ()  [unwired: 1 out]
                n390 = local write "Slide 18"(w410) -> ()
                n391 = local write "Slide 17"(w410) -> ()
              }
            }
          }
          frame True {
            n392 = for {
              N: 55 -> [_]
              i -> [w418]
              stop <- w415 stop-if-true
              n393 = Multiply(x=w418, y=2) -> (x*y=w413:i32)
              "Slide 18" <- w413
              "Slide 17" <- w413
              n394 = Equal?(x=w413, y=99) -> (x = y?=w415:bool)
              n395 = Wait (ms)(milliseconds to wait=u32 50) -> ()  [unwired: 1 out]
            }
          }
        }
      }
      frame "29" {
        n396 = Type Cast(type=TRUE, x=w420) -> (*(type *) &x=w419:bool)
        n397 = case shown="False" w419 {
          frame False {
            n398 = stacked-sequence {
              frame #0 {
                w422 = u8 100 ("Horizontal Progress Bar 2")
                n399 = Wait (ms)(milliseconds to wait=u32 100) -> ()  [unwired: 1 out]
                n400 = local write "Slide 19"(w422) -> ()
                n401 = local write "Slide 20"(w422) -> ()
              }
              frame #1 {
                w424 = u8 90 ("Horizontal Progress Bar 2")
                n402 = Wait (ms)(milliseconds to wait=u32 100) -> ()  [unwired: 1 out]
                n403 = local write "Slide 19"(w424) -> ()
                n404 = local write "Slide 20"(w424) -> ()
              }
              frame #2 {
                w426 = u8 80 ("Horizontal Progress Bar 2")
                n405 = Wait (ms)(milliseconds to wait=u32 100) -> ()  [unwired: 1 out]
                n406 = local write "Slide 19"(w426) -> ()
                n407 = local write "Slide 20"(w426) -> ()
              }
              frame #3 {
                w428 = u8 70 ("Horizontal Progress Bar 2")
                n408 = Wait (ms)(milliseconds to wait=u32 100) -> ()  [unwired: 1 out]
                n409 = local write "Slide 19"(w428) -> ()
                n410 = local write "Slide 20"(w428) -> ()
              }
              frame #4 {
                w430 = u8 60 ("Horizontal Progress Bar 2")
                n411 = Wait (ms)(milliseconds to wait=u32 100) -> ()  [unwired: 1 out]
                n412 = local write "Slide 19"(w430) -> ()
                n413 = local write "Slide 20"(w430) -> ()
              }
              frame #5 {
                w432 = u8 50 ("Horizontal Progress Bar 2")
                n414 = Wait (ms)(milliseconds to wait=u32 100) -> ()  [unwired: 1 out]
                n415 = local write "Slide 19"(w432) -> ()
                n416 = local write "Slide 20"(w432) -> ()
              }
              frame #6 {
                w434 = u8 40 ("Horizontal Progress Bar 2")
                n417 = Wait (ms)(milliseconds to wait=u32 100) -> ()  [unwired: 1 out]
                n418 = local write "Slide 19"(w434) -> ()
                n419 = local write "Slide 20"(w434) -> ()
              }
              frame #7 {
                w436 = u8 30 ("Horizontal Progress Bar 2")
                n420 = Wait (ms)(milliseconds to wait=u32 100) -> ()  [unwired: 1 out]
                n421 = local write "Slide 19"(w436) -> ()
                n422 = local write "Slide 20"(w436) -> ()
              }
              frame #8 {
                w438 = u8 20 ("Horizontal Progress Bar 2")
                n423 = local write "Slide 19"(w438) -> ()
                n424 = local write "Slide 20"(w438) -> ()
                n425 = Wait (ms)(milliseconds to wait=u32 100) -> ()  [unwired: 1 out]
              }
              frame #9 {
                w440 = u8 10 ("Horizontal Progress Bar 2")
                n426 = Wait (ms)(milliseconds to wait=u32 100) -> ()  [unwired: 1 out]
                n427 = local write "Slide 19"(w440) -> ()
                n428 = local write "Slide 20"(w440) -> ()
              }
              frame #10 {
                w442 = u8 0 ("Horizontal Progress Bar 2")
                n429 = Wait (ms)(milliseconds to wait=u32 100) -> ()  [unwired: 1 out]
                n430 = local write "Slide 19"(w442) -> ()
                n431 = local write "Slide 20"(w442) -> ()
              }
            }
          }
          frame True {
            n432 = for {
              N: 55 -> [_]
              i -> [w450]
              stop <- w447 stop-if-true
              n433 = Multiply(x=w450, y=2) -> (x*y=w445:i32)
              "Slide 19" <- w445
              "Slide 20" <- w445
              n434 = Equal?(x=w445, y=99) -> (x = y?=w447:bool)
              n435 = Wait (ms)(milliseconds to wait=u32 50) -> ()  [unwired: 1 out]
            }
          }
        }
      }
      frame "30" {
        n436 = Type Cast(type=TRUE, x=w451) -> (*(type *) &x=w452:bool)
        n437 = case shown="False" w452 {
          frame False {
            n438 = stacked-sequence {
              frame #0 {
                w454 = u8 100 ("Horizontal Progress Bar 2")
                n439 = Wait (ms)(milliseconds to wait=u32 100) -> ()  [unwired: 1 out]
                n440 = local write "Slide 21"(w454) -> ()
                n441 = local write "Slide 22"(w454) -> ()
              }
              frame #1 {
                w456 = u8 90 ("Horizontal Progress Bar 2")
                n442 = Wait (ms)(milliseconds to wait=u32 100) -> ()  [unwired: 1 out]
                n443 = local write "Slide 21"(w456) -> ()
                n444 = local write "Slide 22"(w456) -> ()
              }
              frame #2 {
                w458 = u8 80 ("Horizontal Progress Bar 2")
                n445 = Wait (ms)(milliseconds to wait=u32 100) -> ()  [unwired: 1 out]
                n446 = local write "Slide 21"(w458) -> ()
                n447 = local write "Slide 22"(w458) -> ()
              }
              frame #3 {
                w460 = u8 70 ("Horizontal Progress Bar 2")
                n448 = Wait (ms)(milliseconds to wait=u32 100) -> ()  [unwired: 1 out]
                n449 = local write "Slide 21"(w460) -> ()
                n450 = local write "Slide 22"(w460) -> ()
              }
              frame #4 {
                w462 = u8 60 ("Horizontal Progress Bar 2")
                n451 = local write "Slide 21"(w462) -> ()
                n452 = local write "Slide 22"(w462) -> ()
                n453 = Wait (ms)(milliseconds to wait=u32 100) -> ()  [unwired: 1 out]
              }
              frame #5 {
                w464 = u8 50 ("Horizontal Progress Bar 2")
                n454 = local write "Slide 21"(w464) -> ()
                n455 = Wait (ms)(milliseconds to wait=u32 100) -> ()  [unwired: 1 out]
                n456 = local write "Slide 22"(w464) -> ()
              }
              frame #6 {
                w466 = u8 40 ("Horizontal Progress Bar 2")
                n457 = Wait (ms)(milliseconds to wait=u32 100) -> ()  [unwired: 1 out]
                n458 = local write "Slide 21"(w466) -> ()
                n459 = local write "Slide 22"(w466) -> ()
              }
              frame #7 {
                w468 = u8 30 ("Horizontal Progress Bar 2")
                n460 = Wait (ms)(milliseconds to wait=u32 100) -> ()  [unwired: 1 out]
                n461 = local write "Slide 21"(w468) -> ()
                n462 = local write "Slide 22"(w468) -> ()
              }
              frame #8 {
                w470 = u8 20 ("Horizontal Progress Bar 2")
                n463 = local write "Slide 21"(w470) -> ()
                n464 = local write "Slide 22"(w470) -> ()
                n465 = Wait (ms)(milliseconds to wait=u32 100) -> ()  [unwired: 1 out]
              }
              frame #9 {
                w472 = u8 10 ("Horizontal Progress Bar 2")
                n466 = Wait (ms)(milliseconds to wait=u32 100) -> ()  [unwired: 1 out]
                n467 = local write "Slide 21"(w472) -> ()
                n468 = local write "Slide 22"(w472) -> ()
              }
              frame #10 {
                w474 = u8 0 ("Horizontal Progress Bar 2")
                n469 = Wait (ms)(milliseconds to wait=u32 100) -> ()  [unwired: 1 out]
                n470 = local write "Slide 21"(w474) -> ()
                n471 = local write "Slide 22"(w474) -> ()
              }
            }
          }
          frame True {
            n472 = for {
              N: 55 -> [_]
              i -> [w482]
              stop <- w479 stop-if-true
              n473 = Multiply(x=w482, y=2) -> (x*y=w477:i32)
              "Slide 21" <- w477
              "Slide 22" <- w477
              n474 = Equal?(x=w477, y=99) -> (x = y?=w479:bool)
              n475 = Wait (ms)(milliseconds to wait=u32 50) -> ()  [unwired: 1 out]
            }
          }
        }
      }
      frame "31" {
        n476 = Type Cast(type=TRUE, x=w483) -> (*(type *) &x=w484:bool)
        n477 = case shown="False" w484 {
          frame False {
            n478 = stacked-sequence {
              frame #0 {
                w486 = u8 100 ("Horizontal Progress Bar 2")
                n479 = Wait (ms)(milliseconds to wait=u32 100) -> ()  [unwired: 1 out]
                n480 = local write "Slide 24"(w486) -> ()
                n481 = local write "Slide 23"(w486) -> ()
              }
              frame #1 {
                w488 = u8 90 ("Horizontal Progress Bar 2")
                n482 = Wait (ms)(milliseconds to wait=u32 100) -> ()  [unwired: 1 out]
                n483 = local write "Slide 24"(w488) -> ()
                n484 = local write "Slide 23"(w488) -> ()
              }
              frame #2 {
                w490 = u8 80 ("Horizontal Progress Bar 2")
                n485 = Wait (ms)(milliseconds to wait=u32 100) -> ()  [unwired: 1 out]
                n486 = local write "Slide 24"(w490) -> ()
                n487 = local write "Slide 23"(w490) -> ()
              }
              frame #3 {
                w492 = u8 70 ("Horizontal Progress Bar 2")
                n488 = Wait (ms)(milliseconds to wait=u32 100) -> ()  [unwired: 1 out]
                n489 = local write "Slide 24"(w492) -> ()
                n490 = local write "Slide 23"(w492) -> ()
              }
              frame #4 {
                w494 = u8 60 ("Horizontal Progress Bar 2")
                n491 = Wait (ms)(milliseconds to wait=u32 100) -> ()  [unwired: 1 out]
                n492 = local write "Slide 24"(w494) -> ()
                n493 = local write "Slide 23"(w494) -> ()
              }
              frame #5 {
                w496 = u8 50 ("Horizontal Progress Bar 2")
                n494 = Wait (ms)(milliseconds to wait=u32 100) -> ()  [unwired: 1 out]
                n495 = local write "Slide 24"(w496) -> ()
                n496 = local write "Slide 23"(w496) -> ()
              }
              frame #6 {
                w498 = u8 40 ("Horizontal Progress Bar 2")
                n497 = Wait (ms)(milliseconds to wait=u32 100) -> ()  [unwired: 1 out]
                n498 = local write "Slide 24"(w498) -> ()
                n499 = local write "Slide 23"(w498) -> ()
              }
              frame #7 {
                w500 = u8 30 ("Horizontal Progress Bar 2")
                n500 = Wait (ms)(milliseconds to wait=u32 100) -> ()  [unwired: 1 out]
                n501 = local write "Slide 24"(w500) -> ()
                n502 = local write "Slide 23"(w500) -> ()
              }
              frame #8 {
                w502 = u8 20 ("Horizontal Progress Bar 2")
                n503 = Wait (ms)(milliseconds to wait=u32 100) -> ()  [unwired: 1 out]
                n504 = local write "Slide 24"(w502) -> ()
                n505 = local write "Slide 23"(w502) -> ()
              }
              frame #9 {
                w504 = u8 10 ("Horizontal Progress Bar 2")
                n506 = Wait (ms)(milliseconds to wait=u32 100) -> ()  [unwired: 1 out]
                n507 = local write "Slide 24"(w504) -> ()
                n508 = local write "Slide 23"(w504) -> ()
              }
              frame #10 {
                w506 = u8 0 ("Horizontal Progress Bar 2")
                n509 = Wait (ms)(milliseconds to wait=u32 100) -> ()  [unwired: 1 out]
                n510 = local write "Slide 24"(w506) -> ()
                n511 = local write "Slide 23"(w506) -> ()
              }
            }
          }
          frame True {
            n512 = for {
              N: 55 -> [_]
              i -> [w514]
              stop <- w511 stop-if-true
              n513 = Multiply(x=w514, y=2) -> (x*y=w509:i32)
              "Slide 24" <- w509
              "Slide 23" <- w509
              n514 = Equal?(x=w509, y=99) -> (x = y?=w511:bool)
              n515 = Wait (ms)(milliseconds to wait=u32 50) -> ()  [unwired: 1 out]
            }
          }
        }
      }
      frame "32" {
        n516 = Type Cast(type=TRUE, x=w516) -> (*(type *) &x=→"Boolean 38":bool)
      }
      frame "33" {
        n517 = Type Cast(type=TRUE, x=w519) -> (*(type *) &x=→"Boolean 39":bool)
      }
      frame "34" {
        n518 = Type Cast(type=TRUE, x=w522) -> (*(type *) &x=→"Boolean 43":bool)
      }
      frame "35" {
        n519 = Type Cast(type=TRUE, x=w525) -> (*(type *) &x=→"Boolean 40":bool)
      }
      frame "36" {
        n520 = Type Cast(type=TRUE, x=w528) -> (*(type *) &x=→"Boolean 44":bool)
      }
      frame "37" {
        n521 = Type Cast(type=TRUE, x=w531) -> (*(type *) &x=→"Boolean 41" →"Boolean 42":bool)
      }
      frame "38" {
        n522 = Type Cast(type=TRUE, x=w534) -> (*(type *) &x=→"Boolean 27":bool)
      }
      frame "39" {
        n523 = Type Cast(type=TRUE, x=w537) -> (*(type *) &x=→"Boolean 28":bool)
      }
      frame "40" {
        n524 = Type Cast(type=TRUE, x=w540) -> (*(type *) &x=→"Boolean 29":bool)
      }
      frame "41" {
        n525 = Type Cast(type=TRUE, x=w543) -> (*(type *) &x=→"Boolean 30":bool)
      }
      frame "42" {
        n526 = Type Cast(type=TRUE, x=w546) -> (*(type *) &x=→"Boolean 31":bool)
      }
      frame "43" {
        n527 = Type Cast(type=TRUE, x=w549) -> (*(type *) &x=→"Boolean 32":bool)
      }
      frame "44" {
        n528 = Type Cast(type=TRUE, x=w552) -> (*(type *) &x=→"Boolean 33":bool)
      }
      frame "45" {
        n529 = Type Cast(type=TRUE, x=w555) -> (*(type *) &x=→"Boolean 34" →"Boolean 35" →"Boolean 36" →"Boolean 37":bool)
      }
      frame "46" {
        n530 = In Range and Coerce(upper limit="17", x=w559, lower limit="12") -> (In Range?=w557:bool)  [unwired: 1 out]
        n531 = case shown="True" w557 {
          frame False {
            w564 = 20 ("Thermometer")
            w565 = FALSE
            n532 = local write "Boolean 46"(w565) -> ()
            n533 = local write "Boolean 49"(w565) -> ()
            n534 = local write "Boolean 50"(w565) -> ()
            n535 = local write "Boolean 45"(w565) -> ()
            n536 = local write "MasterRoom Temprature"(w564) -> ()
            n537 = local write "LivingRoom2 Temprature"(w564) -> ()
            n538 = local write "LivingRoom Temprature"(w564) -> ()
            n539 = local write "DiningRoom Temprature"(w564) -> ()
            n540 = local write "Bedroom2 Temprature"(w564) -> ()
            n541 = local write "Bedroom Temprature"(w564) -> ()
            n542 = local write "Boolean 47"(w565) -> ()
            n543 = local write "Boolean 48"(w565) -> ()
          }
          frame True {
            w566 = TRUE
            n544 = stacked-sequence {
              frame #0 {
                n545 = for {
                  N: 18 -> [_]
                  i -> [w570]
                  n546 = Wait (ms)(milliseconds to wait=u32 60) -> ()  [unwired: 1 out]
                  n547 = Multiply(x=w570, y=2) -> (x*y=→"Bedroom Temprature" →"MasterRoom Temprature" →"DiningRoom Temprature" →"Bedroom2 Temprature" →"LivingRoom2 Temprature" →"LivingRoom Temprature":i32)
                }
              }
              frame #1 {
                w573 = 35 ("Thermometer")
                n548 = local write "MasterRoom Temprature"(w573) -> ()
                n549 = local write "LivingRoom2 Temprature"(w573) -> ()
                n550 = local write "LivingRoom Temprature"(w573) -> ()
                n551 = local write "DiningRoom Temprature"(w573) -> ()
                n552 = local write "Bedroom2 Temprature"(w573) -> ()
                n553 = local write "Bedroom Temprature"(w573) -> ()
                n554 = Wait (ms)(milliseconds to wait=u32 1000) -> ()  [unwired: 1 out]
              }
              frame #2 {
                w575 = 34 ("Thermometer")
                n555 = local write "MasterRoom Temprature"(w575) -> ()
                n556 = local write "LivingRoom2 Temprature"(w575) -> ()
                n557 = local write "LivingRoom Temprature"(w575) -> ()
                n558 = local write "DiningRoom Temprature"(w575) -> ()
                n559 = local write "Bedroom2 Temprature"(w575) -> ()
                n560 = local write "Bedroom Temprature"(w575) -> ()
                n561 = Wait (ms)(milliseconds to wait=u32 1000) -> ()  [unwired: 1 out]
              }
              frame #3 {
                w577 = 32 ("Thermometer")
                n562 = local write "MasterRoom Temprature"(w577) -> ()
                n563 = local write "LivingRoom2 Temprature"(w577) -> ()
                n564 = local write "LivingRoom Temprature"(w577) -> ()
                n565 = local write "DiningRoom Temprature"(w577) -> ()
                n566 = local write "Bedroom2 Temprature"(w577) -> ()
                n567 = local write "Bedroom Temprature"(w577) -> ()
                n568 = Wait (ms)(milliseconds to wait=u32 1000) -> ()  [unwired: 1 out]
              }
              frame #4 {
                w579 = 30 ("Thermometer")
                n569 = local write "MasterRoom Temprature"(w579) -> ()
                n570 = local write "LivingRoom2 Temprature"(w579) -> ()
                n571 = local write "LivingRoom Temprature"(w579) -> ()
                n572 = local write "DiningRoom Temprature"(w579) -> ()
                n573 = local write "Bedroom2 Temprature"(w579) -> ()
                n574 = local write "Bedroom Temprature"(w579) -> ()
                n575 = Wait (ms)(milliseconds to wait=u32 1000) -> ()  [unwired: 1 out]
              }
              frame #5 {
                w581 = 28 ("Thermometer")
                n576 = local write "MasterRoom Temprature"(w581) -> ()
                n577 = local write "LivingRoom2 Temprature"(w581) -> ()
                n578 = local write "LivingRoom Temprature"(w581) -> ()
                n579 = local write "DiningRoom Temprature"(w581) -> ()
                n580 = local write "Bedroom2 Temprature"(w581) -> ()
                n581 = local write "Bedroom Temprature"(w581) -> ()
                n582 = Wait (ms)(milliseconds to wait=u32 1000) -> ()  [unwired: 1 out]
              }
              frame #6 {
                w583 = 26 ("Thermometer")
                n583 = local write "MasterRoom Temprature"(w583) -> ()
                n584 = local write "LivingRoom2 Temprature"(w583) -> ()
                n585 = local write "LivingRoom Temprature"(w583) -> ()
                n586 = local write "DiningRoom Temprature"(w583) -> ()
                n587 = local write "Bedroom2 Temprature"(w583) -> ()
                n588 = local write "Bedroom Temprature"(w583) -> ()
                n589 = Wait (ms)(milliseconds to wait=u32 1000) -> ()  [unwired: 1 out]
              }
              frame #7 {
                w585 = 24 ("Thermometer")
                n590 = local write "MasterRoom Temprature"(w585) -> ()
                n591 = local write "LivingRoom2 Temprature"(w585) -> ()
                n592 = local write "LivingRoom Temprature"(w585) -> ()
                n593 = local write "DiningRoom Temprature"(w585) -> ()
                n594 = local write "Bedroom2 Temprature"(w585) -> ()
                n595 = local write "Bedroom Temprature"(w585) -> ()
                n596 = Wait (ms)(milliseconds to wait=u32 1000) -> ()  [unwired: 1 out]
              }
              frame #8 {
                w587 = 22 ("Thermometer")
                n597 = local write "MasterRoom Temprature"(w587) -> ()
                n598 = local write "LivingRoom2 Temprature"(w587) -> ()
                n599 = local write "LivingRoom Temprature"(w587) -> ()
                n600 = local write "DiningRoom Temprature"(w587) -> ()
                n601 = local write "Bedroom2 Temprature"(w587) -> ()
                n602 = local write "Bedroom Temprature"(w587) -> ()
                n603 = Wait (ms)(milliseconds to wait=u32 1000) -> ()  [unwired: 1 out]
              }
              frame #9 {
                w588 = 20 ("Thermometer")
                n604 = local write "MasterRoom Temprature"(w588) -> ()
                n605 = local write "LivingRoom2 Temprature"(w588) -> ()
                n606 = local write "LivingRoom Temprature"(w588) -> ()
                n607 = local write "DiningRoom Temprature"(w588) -> ()
                n608 = local write "Bedroom2 Temprature"(w588) -> ()
                n609 = local write "Bedroom Temprature"(w588) -> ()
              }
            }
            "Boolean 47" <- w566
            "Boolean 46" <- w566
            "Boolean 48" <- w566
            "Boolean 50" <- w566
            "Boolean 49" <- w566
            "Boolean 45" <- w566
          }
        }
        n610 = In Range and Coerce(upper limit="18", x=w559, lower limit="06") -> (In Range?=w558:bool)  [unwired: 1 out]
        n611 = case shown="False" w558 {
          frame False {
            w589 = TRUE
            n612 = local write "Boolean 4"(w589) -> ()
            n613 = local write "Boolean 5"(w589) -> ()
            n614 = local write "Boolean 36"(w589) -> ()
            n615 = local write "Boolean 37"(w589) -> ()
            n616 = local write "Boolean 2"(w589) -> ()
            n617 = local write "Boolean 34"(w589) -> ()
            n618 = local write "Boolean 35"(w589) -> ()
            n619 = local write "Boolean 3"(w589) -> ()
            n620 = local write "Boolean 33"(w589) -> ()
            n621 = local write "Boolean"(w589) -> ()
            n622 = local write "Boolean 14"(w589) -> ()
            n623 = local write "Boolean 15"(w589) -> ()
            n624 = local write "Boolean 16"(w589) -> ()
            n625 = local write "Boolean 12"(w589) -> ()
            n626 = local write "Boolean 6"(w589) -> ()
            n627 = local write "Boolean 7"(w589) -> ()
            n628 = local write "Boolean 13"(w589) -> ()
            n629 = local write "Boolean 10"(w589) -> ()
            n630 = local write "Boolean 11"(w589) -> ()
            n631 = local write "Boolean 8"(w589) -> ()
            n632 = local write "Boolean 31"(w589) -> ()
            n633 = local write "Boolean 9"(w589) -> ()
            n634 = local write "Boolean 32"(w589) -> ()
            n635 = local write "Boolean 28"(w589) -> ()
            n636 = local write "Boolean 29"(w589) -> ()
            n637 = local write "Boolean 30"(w589) -> ()
            n638 = local write "Boolean 27"(w589) -> ()
            n639 = for {
              N: 55 -> [_]
              i -> [w595]
              stop <- w592 stop-if-true
              n640 = Wait (ms)(milliseconds to wait=u32 50) -> ()  [unwired: 1 out]
              n641 = Multiply(x=w595, y=2) -> (x*y=w591:i32)
              n642 = Equal?(x=w591, y=99) -> (x = y?=w592:bool)
              n643 = local write "Slide 4"(w591) -> ()
              n644 = local write "Slide 3"(w591) -> ()
              n645 = local write "Slide 2"(w591) -> ()
              n646 = local write "Slide"(w591) -> ()
              n647 = local write "Slide 10"(w591) -> ()
              n648 = local write "Slide 5"(w591) -> ()
              n649 = local write "Slide 6"(w591) -> ()
              n650 = local write "Slide 7"(w591) -> ()
              n651 = local write "Slide 15"(w591) -> ()
              n652 = local write "Slide 8"(w591) -> ()
              n653 = local write "Slide 11"(w591) -> ()
              n654 = local write "Slide 13"(w591) -> ()
              n655 = local write "Slide 12"(w591) -> ()
              n656 = local write "Slide 14"(w591) -> ()
              n657 = local write "Slide 21"(w591) -> ()
              n658 = local write "Slide 18"(w591) -> ()
              n659 = local write "Slide 19"(w591) -> ()
              n660 = local write "Slide 20"(w591) -> ()
              n661 = local write "Slide 22"(w591) -> ()
              n662 = local write "Slide 24"(w591) -> ()
              n663 = local write "Slide 9"(w591) -> ()
              n664 = local write "Slide 16"(w591) -> ()
              n665 = local write "Slide 17"(w591) -> ()
              n666 = local write "Slide 23"(w591) -> ()
            }
          }
          frame True {
            w597 = FALSE
            n667 = stacked-sequence {
              frame #0 {
                w598 = u8 100 ("Horizontal Progress Bar 2")
                n668 = Wait (ms)(milliseconds to wait=u32 100) -> ()  [unwired: 1 out]
                n669 = local write "Slide 4"(w598) -> ()
                n670 = local write "Slide 3"(w598) -> ()
                n671 = local write "Slide 2"(w598) -> ()
                n672 = local write "Slide"(w598) -> ()
                n673 = local write "Slide 10"(w598) -> ()
                n674 = local write "Slide 5"(w598) -> ()
                n675 = local write "Slide 6"(w598) -> ()
                n676 = local write "Slide 7"(w598) -> ()
                n677 = local write "Slide 15"(w598) -> ()
                n678 = local write "Slide 8"(w598) -> ()
                n679 = local write "Slide 11"(w598) -> ()
                n680 = local write "Slide 13"(w598) -> ()
                n681 = local write "Slide 12"(w598) -> ()
                n682 = local write "Slide 14"(w598) -> ()
                n683 = local write "Slide 21"(w598) -> ()
                n684 = local write "Slide 18"(w598) -> ()
                n685 = local write "Slide 19"(w598) -> ()
                n686 = local write "Slide 20"(w598) -> ()
                n687 = local write "Slide 22"(w598) -> ()
                n688 = local write "Slide 24"(w598) -> ()
                n689 = local write "Slide 16"(w598) -> ()
                n690 = local write "Slide 17"(w598) -> ()
                n691 = local write "Slide 23"(w598) -> ()
                n692 = local write "Slide 9"(w598) -> ()
              }
              frame #1 {
                w600 = u8 90 ("Horizontal Progress Bar 2")
                n693 = Wait (ms)(milliseconds to wait=u32 100) -> ()  [unwired: 1 out]
                n694 = local write "Slide 4"(w600) -> ()
                n695 = local write "Slide 3"(w600) -> ()
                n696 = local write "Slide 2"(w600) -> ()
                n697 = local write "Slide"(w600) -> ()
                n698 = local write "Slide 10"(w600) -> ()
                n699 = local write "Slide 5"(w600) -> ()
                n700 = local write "Slide 6"(w600) -> ()
                n701 = local write "Slide 7"(w600) -> ()
                n702 = local write "Slide 15"(w600) -> ()
                n703 = local write "Slide 8"(w600) -> ()
                n704 = local write "Slide 11"(w600) -> ()
                n705 = local write "Slide 13"(w600) -> ()
                n706 = local write "Slide 12"(w600) -> ()
                n707 = local write "Slide 14"(w600) -> ()
                n708 = local write "Slide 21"(w600) -> ()
                n709 = local write "Slide 18"(w600) -> ()
                n710 = local write "Slide 19"(w600) -> ()
                n711 = local write "Slide 20"(w600) -> ()
                n712 = local write "Slide 22"(w600) -> ()
                n713 = local write "Slide 24"(w600) -> ()
                n714 = local write "Slide 16"(w600) -> ()
                n715 = local write "Slide 17"(w600) -> ()
                n716 = local write "Slide 23"(w600) -> ()
                n717 = local write "Slide 9"(w600) -> ()
              }
              frame #2 {
                w602 = u8 80 ("Horizontal Progress Bar 2")
                n718 = Wait (ms)(milliseconds to wait=u32 100) -> ()  [unwired: 1 out]
                n719 = local write "Slide 4"(w602) -> ()
                n720 = local write "Slide 3"(w602) -> ()
                n721 = local write "Slide 2"(w602) -> ()
                n722 = local write "Slide"(w602) -> ()
                n723 = local write "Slide 10"(w602) -> ()
                n724 = local write "Slide 5"(w602) -> ()
                n725 = local write "Slide 6"(w602) -> ()
                n726 = local write "Slide 7"(w602) -> ()
                n727 = local write "Slide 15"(w602) -> ()
                n728 = local write "Slide 8"(w602) -> ()
                n729 = local write "Slide 11"(w602) -> ()
                n730 = local write "Slide 13"(w602) -> ()
                n731 = local write "Slide 12"(w602) -> ()
                n732 = local write "Slide 14"(w602) -> ()
                n733 = local write "Slide 21"(w602) -> ()
                n734 = local write "Slide 18"(w602) -> ()
                n735 = local write "Slide 19"(w602) -> ()
                n736 = local write "Slide 20"(w602) -> ()
                n737 = local write "Slide 22"(w602) -> ()
                n738 = local write "Slide 24"(w602) -> ()
                n739 = local write "Slide 16"(w602) -> ()
                n740 = local write "Slide 17"(w602) -> ()
                n741 = local write "Slide 23"(w602) -> ()
                n742 = local write "Slide 9"(w602) -> ()
              }
              frame #3 {
                w604 = u8 70 ("Horizontal Progress Bar 2")
                n743 = Wait (ms)(milliseconds to wait=u32 100) -> ()  [unwired: 1 out]
                n744 = local write "Slide 4"(w604) -> ()
                n745 = local write "Slide 3"(w604) -> ()
                n746 = local write "Slide 2"(w604) -> ()
                n747 = local write "Slide"(w604) -> ()
                n748 = local write "Slide 10"(w604) -> ()
                n749 = local write "Slide 5"(w604) -> ()
                n750 = local write "Slide 6"(w604) -> ()
                n751 = local write "Slide 7"(w604) -> ()
                n752 = local write "Slide 15"(w604) -> ()
                n753 = local write "Slide 8"(w604) -> ()
                n754 = local write "Slide 11"(w604) -> ()
                n755 = local write "Slide 13"(w604) -> ()
                n756 = local write "Slide 12"(w604) -> ()
                n757 = local write "Slide 14"(w604) -> ()
                n758 = local write "Slide 21"(w604) -> ()
                n759 = local write "Slide 18"(w604) -> ()
                n760 = local write "Slide 19"(w604) -> ()
                n761 = local write "Slide 20"(w604) -> ()
                n762 = local write "Slide 22"(w604) -> ()
                n763 = local write "Slide 24"(w604) -> ()
                n764 = local write "Slide 16"(w604) -> ()
                n765 = local write "Slide 17"(w604) -> ()
                n766 = local write "Slide 23"(w604) -> ()
                n767 = local write "Slide 9"(w604) -> ()
              }
              frame #4 {
                w606 = u8 60 ("Horizontal Progress Bar 2")
                n768 = Wait (ms)(milliseconds to wait=u32 100) -> ()  [unwired: 1 out]
                n769 = local write "Slide 4"(w606) -> ()
                n770 = local write "Slide 3"(w606) -> ()
                n771 = local write "Slide 2"(w606) -> ()
                n772 = local write "Slide"(w606) -> ()
                n773 = local write "Slide 10"(w606) -> ()
                n774 = local write "Slide 5"(w606) -> ()
                n775 = local write "Slide 6"(w606) -> ()
                n776 = local write "Slide 7"(w606) -> ()
                n777 = local write "Slide 15"(w606) -> ()
                n778 = local write "Slide 8"(w606) -> ()
                n779 = local write "Slide 11"(w606) -> ()
                n780 = local write "Slide 13"(w606) -> ()
                n781 = local write "Slide 12"(w606) -> ()
                n782 = local write "Slide 14"(w606) -> ()
                n783 = local write "Slide 21"(w606) -> ()
                n784 = local write "Slide 18"(w606) -> ()
                n785 = local write "Slide 19"(w606) -> ()
                n786 = local write "Slide 20"(w606) -> ()
                n787 = local write "Slide 22"(w606) -> ()
                n788 = local write "Slide 24"(w606) -> ()
                n789 = local write "Slide 16"(w606) -> ()
                n790 = local write "Slide 17"(w606) -> ()
                n791 = local write "Slide 23"(w606) -> ()
                n792 = local write "Slide 9"(w606) -> ()
              }
              frame #5 {
                w608 = u8 50 ("Horizontal Progress Bar 2")
                n793 = Wait (ms)(milliseconds to wait=u32 100) -> ()  [unwired: 1 out]
                n794 = local write "Slide 4"(w608) -> ()
                n795 = local write "Slide 3"(w608) -> ()
                n796 = local write "Slide 2"(w608) -> ()
                n797 = local write "Slide"(w608) -> ()
                n798 = local write "Slide 10"(w608) -> ()
                n799 = local write "Slide 5"(w608) -> ()
                n800 = local write "Slide 6"(w608) -> ()
                n801 = local write "Slide 7"(w608) -> ()
                n802 = local write "Slide 15"(w608) -> ()
                n803 = local write "Slide 8"(w608) -> ()
                n804 = local write "Slide 11"(w608) -> ()
                n805 = local write "Slide 13"(w608) -> ()
                n806 = local write "Slide 12"(w608) -> ()
                n807 = local write "Slide 14"(w608) -> ()
                n808 = local write "Slide 21"(w608) -> ()
                n809 = local write "Slide 18"(w608) -> ()
                n810 = local write "Slide 19"(w608) -> ()
                n811 = local write "Slide 20"(w608) -> ()
                n812 = local write "Slide 22"(w608) -> ()
                n813 = local write "Slide 24"(w608) -> ()
                n814 = local write "Slide 16"(w608) -> ()
                n815 = local write "Slide 17"(w608) -> ()
                n816 = local write "Slide 23"(w608) -> ()
                n817 = local write "Slide 9"(w608) -> ()
              }
              frame #6 {
                w610 = u8 40 ("Horizontal Progress Bar 2")
                n818 = Wait (ms)(milliseconds to wait=u32 100) -> ()  [unwired: 1 out]
                n819 = local write "Slide 4"(w610) -> ()
                n820 = local write "Slide 3"(w610) -> ()
                n821 = local write "Slide 2"(w610) -> ()
                n822 = local write "Slide"(w610) -> ()
                n823 = local write "Slide 10"(w610) -> ()
                n824 = local write "Slide 5"(w610) -> ()
                n825 = local write "Slide 6"(w610) -> ()
                n826 = local write "Slide 7"(w610) -> ()
                n827 = local write "Slide 15"(w610) -> ()
                n828 = local write "Slide 8"(w610) -> ()
                n829 = local write "Slide 11"(w610) -> ()
                n830 = local write "Slide 13"(w610) -> ()
                n831 = local write "Slide 12"(w610) -> ()
                n832 = local write "Slide 14"(w610) -> ()
                n833 = local write "Slide 21"(w610) -> ()
                n834 = local write "Slide 18"(w610) -> ()
                n835 = local write "Slide 19"(w610) -> ()
                n836 = local write "Slide 20"(w610) -> ()
                n837 = local write "Slide 22"(w610) -> ()
                n838 = local write "Slide 24"(w610) -> ()
                n839 = local write "Slide 16"(w610) -> ()
                n840 = local write "Slide 17"(w610) -> ()
                n841 = local write "Slide 23"(w610) -> ()
                n842 = local write "Slide 9"(w610) -> ()
              }
              frame #7 {
                w612 = u8 30 ("Horizontal Progress Bar 2")
                n843 = Wait (ms)(milliseconds to wait=u32 100) -> ()  [unwired: 1 out]
                n844 = local write "Slide 4"(w612) -> ()
                n845 = local write "Slide 3"(w612) -> ()
                n846 = local write "Slide 2"(w612) -> ()
                n847 = local write "Slide"(w612) -> ()
                n848 = local write "Slide 10"(w612) -> ()
                n849 = local write "Slide 5"(w612) -> ()
                n850 = local write "Slide 6"(w612) -> ()
                n851 = local write "Slide 7"(w612) -> ()
                n852 = local write "Slide 15"(w612) -> ()
                n853 = local write "Slide 8"(w612) -> ()
                n854 = local write "Slide 11"(w612) -> ()
                n855 = local write "Slide 13"(w612) -> ()
                n856 = local write "Slide 12"(w612) -> ()
                n857 = local write "Slide 14"(w612) -> ()
                n858 = local write "Slide 21"(w612) -> ()
                n859 = local write "Slide 18"(w612) -> ()
                n860 = local write "Slide 19"(w612) -> ()
                n861 = local write "Slide 20"(w612) -> ()
                n862 = local write "Slide 22"(w612) -> ()
                n863 = local write "Slide 24"(w612) -> ()
                n864 = local write "Slide 16"(w612) -> ()
                n865 = local write "Slide 17"(w612) -> ()
                n866 = local write "Slide 23"(w612) -> ()
                n867 = local write "Slide 9"(w612) -> ()
              }
              frame #8 {
                w614 = u8 20 ("Horizontal Progress Bar 2")
                n868 = Wait (ms)(milliseconds to wait=u32 100) -> ()  [unwired: 1 out]
                n869 = local write "Slide 4"(w614) -> ()
                n870 = local write "Slide 3"(w614) -> ()
                n871 = local write "Slide 2"(w614) -> ()
                n872 = local write "Slide"(w614) -> ()
                n873 = local write "Slide 10"(w614) -> ()
                n874 = local write "Slide 5"(w614) -> ()
                n875 = local write "Slide 6"(w614) -> ()
                n876 = local write "Slide 7"(w614) -> ()
                n877 = local write "Slide 15"(w614) -> ()
                n878 = local write "Slide 8"(w614) -> ()
                n879 = local write "Slide 11"(w614) -> ()
                n880 = local write "Slide 13"(w614) -> ()
                n881 = local write "Slide 12"(w614) -> ()
                n882 = local write "Slide 14"(w614) -> ()
                n883 = local write "Slide 21"(w614) -> ()
                n884 = local write "Slide 18"(w614) -> ()
                n885 = local write "Slide 19"(w614) -> ()
                n886 = local write "Slide 20"(w614) -> ()
                n887 = local write "Slide 22"(w614) -> ()
                n888 = local write "Slide 24"(w614) -> ()
                n889 = local write "Slide 16"(w614) -> ()
                n890 = local write "Slide 17"(w614) -> ()
                n891 = local write "Slide 23"(w614) -> ()
                n892 = local write "Slide 9"(w614) -> ()
              }
              frame #9 {
                w616 = u8 10 ("Horizontal Progress Bar 2")
                n893 = Wait (ms)(milliseconds to wait=u32 100) -> ()  [unwired: 1 out]
                n894 = local write "Slide 4"(w616) -> ()
                n895 = local write "Slide 3"(w616) -> ()
                n896 = local write "Slide 2"(w616) -> ()
                n897 = local write "Slide"(w616) -> ()
                n898 = local write "Slide 10"(w616) -> ()
                n899 = local write "Slide 5"(w616) -> ()
                n900 = local write "Slide 6"(w616) -> ()
                n901 = local write "Slide 7"(w616) -> ()
                n902 = local write "Slide 15"(w616) -> ()
                n903 = local write "Slide 8"(w616) -> ()
                n904 = local write "Slide 11"(w616) -> ()
                n905 = local write "Slide 13"(w616) -> ()
                n906 = local write "Slide 12"(w616) -> ()
                n907 = local write "Slide 14"(w616) -> ()
                n908 = local write "Slide 21"(w616) -> ()
                n909 = local write "Slide 18"(w616) -> ()
                n910 = local write "Slide 19"(w616) -> ()
                n911 = local write "Slide 20"(w616) -> ()
                n912 = local write "Slide 22"(w616) -> ()
                n913 = local write "Slide 24"(w616) -> ()
                n914 = local write "Slide 16"(w616) -> ()
                n915 = local write "Slide 17"(w616) -> ()
                n916 = local write "Slide 23"(w616) -> ()
                n917 = local write "Slide 9"(w616) -> ()
              }
              frame #10 {
                w618 = u8 0 ("Horizontal Progress Bar 2")
                n918 = Wait (ms)(milliseconds to wait=u32 100) -> ()  [unwired: 1 out]
                n919 = local write "Slide 4"(w618) -> ()
                n920 = local write "Slide 3"(w618) -> ()
                n921 = local write "Slide 2"(w618) -> ()
                n922 = local write "Slide"(w618) -> ()
                n923 = local write "Slide 10"(w618) -> ()
                n924 = local write "Slide 5"(w618) -> ()
                n925 = local write "Slide 6"(w618) -> ()
                n926 = local write "Slide 7"(w618) -> ()
                n927 = local write "Slide 15"(w618) -> ()
                n928 = local write "Slide 8"(w618) -> ()
                n929 = local write "Slide 11"(w618) -> ()
                n930 = local write "Slide 13"(w618) -> ()
                n931 = local write "Slide 12"(w618) -> ()
                n932 = local write "Slide 14"(w618) -> ()
                n933 = local write "Slide 21"(w618) -> ()
                n934 = local write "Slide 18"(w618) -> ()
                n935 = local write "Slide 19"(w618) -> ()
                n936 = local write "Slide 20"(w618) -> ()
                n937 = local write "Slide 22"(w618) -> ()
                n938 = local write "Slide 24"(w618) -> ()
                n939 = local write "Slide 16"(w618) -> ()
                n940 = local write "Slide 17"(w618) -> ()
                n941 = local write "Slide 23"(w618) -> ()
                n942 = local write "Slide 9"(w618) -> ()
              }
            }
            n943 = local write "Boolean 4"(w597) -> ()
            n944 = local write "Boolean 5"(w597) -> ()
            n945 = local write "Boolean 36"(w597) -> ()
            n946 = local write "Boolean 37"(w597) -> ()
            n947 = local write "Boolean 2"(w597) -> ()
            n948 = local write "Boolean 34"(w597) -> ()
            n949 = local write "Boolean 35"(w597) -> ()
            n950 = local write "Boolean 3"(w597) -> ()
            n951 = local write "Boolean 33"(w597) -> ()
            n952 = local write "Boolean"(w597) -> ()
            n953 = local write "Boolean 14"(w597) -> ()
            n954 = local write "Boolean 15"(w597) -> ()
            n955 = local write "Boolean 16"(w597) -> ()
            n956 = local write "Boolean 12"(w597) -> ()
            n957 = local write "Boolean 6"(w597) -> ()
            n958 = local write "Boolean 7"(w597) -> ()
            n959 = local write "Boolean 13"(w597) -> ()
            n960 = local write "Boolean 31"(w597) -> ()
            n961 = local write "Boolean 10"(w597) -> ()
            n962 = local write "Boolean 11"(w597) -> ()
            n963 = local write "Boolean 8"(w597) -> ()
            n964 = local write "Boolean 9"(w597) -> ()
            n965 = local write "Boolean 32"(w597) -> ()
            n966 = local write "Boolean 28"(w597) -> ()
            n967 = local write "Boolean 29"(w597) -> ()
            n968 = local write "Boolean 30"(w597) -> ()
            n969 = local write "Boolean 27"(w597) -> ()
          }
        }
      }
      frame "47" {
        n970 = property class="IWMPPlayer4"(reference=w623, "URL"="E:\\Breaking Bad Season 2 Extra - Distribution Network.mp4") -> (reference out=w620:refnum<k7>)  [unwired: 1 in, 1 out]
        n971 = property class="IWMPPlayer4"(reference=w620) -> ("controls"=w622:refnum<k7>)  [unwired: 1 in, 2 out]
        n972 = invoke class="IWMPControls" method="play"(reference=w622) -> ()  [unwired: 2 in, 3 out]
      }
      frame "48" {
        n973 = property class="IWMPPlayer4"(reference=w626, "URL"="E:\\Breaking Bad Season 2 Extra - Minisode 03 - Better Call Saul - Badger.mp4") -> (reference out=w624:refnum<k7>)  [unwired: 1 in, 1 out]
        n974 = property class="IWMPPlayer4"(reference=w624) -> ("controls"=w627:refnum<k7>)  [unwired: 1 in, 2 out]
        n975 = invoke class="IWMPControls" method="play"(reference=w627) -> ()  [unwired: 2 in, 3 out]
      }
      frame "49" {
        n976 = property class="IWMPPlayer4"(reference=w628) -> ("controls"=w629:refnum<k7>)  [unwired: 1 in, 2 out]
        n977 = invoke class="IWMPControls" method="play"(reference=w629) -> ()  [unwired: 2 in, 3 out]
      }
      frame "50" {
        n978 = property class="IWMPPlayer4"(reference=w630) -> ("controls"=w631:refnum<k7>)  [unwired: 1 in, 2 out]
        n979 = invoke class="IWMPControls" method="pause"(reference=w631) -> ()  [unwired: 2 in, 3 out]
      }
      frame "51" {
        n980 = property class="IWMPPlayer4"(reference=w632) -> ("controls"=w633:refnum<k7>)  [unwired: 1 in, 2 out]
        n981 = invoke class="IWMPControls" method="stop"(reference=w633) -> ()  [unwired: 2 in, 3 out]
      }
      frame "52" {
        n982 = Type Cast(type=0.0, x=w635) -> (*(type *) &x=w634:dbl)
        n983 = property class="IWMPPlayer4"(reference=w638) -> ("settings"=w637:refnum<k7>)  [unwired: 1 in, 2 out]
        n984 = property class="IWMPSettings"(reference=w637, "volume"=w634) -> ()  [unwired: 1 in, 2 out]
      }
      frame "53" {
        n985 = Type Cast(type=0.0, x=w640) -> (*(type *) &x=w639:dbl)
        n986 = property class="IWMPPlayer4"(reference=w642) -> ("settings"=w643:refnum<k7>)  [unwired: 1 in, 2 out]
        n987 = property class="IWMPSettings"(reference=w643, "volume"=w639) -> ()  [unwired: 1 in, 2 out]
      }
      frame "54" {
        n988 = property class="IWMPPlayer4"(reference=w644) -> ("controls"=w645:refnum<k7>)  [unwired: 1 in, 2 out]
        n989 = invoke class="IWMPControls" method="fastForward"(reference=w645) -> ()  [unwired: 2 in, 3 out]
      }
      frame "55" {
        n990 = property class="IWMPPlayer4"(reference=w646) -> ("controls"=w647:refnum<k7>)  [unwired: 1 in, 2 out]
        n991 = invoke class="IWMPControls" method="fastReverse"(reference=w647) -> ()  [unwired: 2 in, 3 out]
      }
      frame "56" {
        n992 = property class="IWMPPlayer4"(reference=w648) -> ("controls"=w650:refnum<k7>)  [unwired: 1 in, 2 out]
        n993 = property class="IWMPPlayer4"(reference=w648, "URL"="E:\\Breaking Bad Season 2 Extra - Minisode 03 - Better Call Saul - Badger.mp4") -> ()  [unwired: 1 in, 2 out]
        n994 = invoke class="IWMPControls" method="play"(reference=w650) -> ()  [unwired: 2 in, 3 out]
      }
      frame "57" {
        n995 = property class="IWMPPlayer4"(reference=w651) -> ("controls"=w653:refnum<k7>)  [unwired: 1 in, 2 out]
        n996 = property class="IWMPPlayer4"(reference=w651, "URL"="") -> ()  [unwired: 1 in, 2 out]
        n997 = invoke class="IWMPControls" method="stop"(reference=w653) -> ()  [unwired: 2 in, 3 out]
      }
      frame "58" {
        n998 = Type Cast(type=TRUE, x=w654) -> (*(type *) &x=w656:bool)
        n999 = case shown="True" w656 {
          frame False {
            n1000 = stacked-sequence {
              frame #0 {
                n1001 = Wait (ms)(milliseconds to wait=u32 100) -> ()  [unwired: 1 out]
                n1002 = local write "Slide 27"(u8 100 ("Horizontal Progress Bar 2")) -> ()
              }
              frame #1 {
                n1003 = local write "Slide 27"(u8 90 ("Horizontal Progress Bar 2")) -> ()
                n1004 = Wait (ms)(milliseconds to wait=u32 100) -> ()  [unwired: 1 out]
              }
              frame #2 {
                n1005 = Wait (ms)(milliseconds to wait=u32 100) -> ()  [unwired: 1 out]
                n1006 = local write "Slide 27"(u8 80 ("Horizontal Progress Bar 2")) -> ()
              }
              frame #3 {
                n1007 = local write "Slide 27"(u8 70 ("Horizontal Progress Bar 2")) -> ()
                n1008 = Wait (ms)(milliseconds to wait=u32 100) -> ()  [unwired: 1 out]
              }
              frame #4 {
                n1009 = local write "Slide 27"(u8 60 ("Horizontal Progress Bar 2")) -> ()
                n1010 = Wait (ms)(milliseconds to wait=u32 100) -> ()  [unwired: 1 out]
              }
              frame #5 {
                n1011 = local write "Slide 27"(u8 50 ("Horizontal Progress Bar 2")) -> ()
                n1012 = Wait (ms)(milliseconds to wait=u32 100) -> ()  [unwired: 1 out]
              }
              frame #6 {
                n1013 = local write "Slide 27"(u8 40 ("Horizontal Progress Bar 2")) -> ()
                n1014 = Wait (ms)(milliseconds to wait=u32 100) -> ()  [unwired: 1 out]
              }
              frame #7 {
                n1015 = Wait (ms)(milliseconds to wait=u32 100) -> ()  [unwired: 1 out]
                n1016 = local write "Slide 27"(u8 30 ("Horizontal Progress Bar 2")) -> ()
              }
              frame #8 {
                n1017 = local write "Slide 27"(u8 20 ("Horizontal Progress Bar 2")) -> ()
                n1018 = Wait (ms)(milliseconds to wait=u32 100) -> ()  [unwired: 1 out]
              }
              frame #9 {
                n1019 = Wait (ms)(milliseconds to wait=u32 100) -> ()  [unwired: 1 out]
                n1020 = local write "Slide 27"(u8 10 ("Horizontal Progress Bar 2")) -> ()
              }
              frame #10 {
                n1021 = local write "Slide 27"(u8 0 ("Horizontal Progress Bar 2")) -> ()
                n1022 = Wait (ms)(milliseconds to wait=u32 100) -> ()  [unwired: 1 out]
              }
            }
          }
          frame True {
            n1023 = for {
              N: 55 -> [_]
              i -> [w685]
              stop <- w682 stop-if-true
              n1024 = Multiply(x=w685, y=2) -> (x*y=w680:i32)
              "Slide 27" <- w680
              n1025 = Equal?(x=w680, y=99) -> (x = y?=w682:bool)
              n1026 = Wait (ms)(milliseconds to wait=u32 50) -> ()  [unwired: 1 out]
            }
          }
        }
      }
      frame "59" {
        n1027 = Type Cast(type=TRUE, x=w686) -> (*(type *) &x=w688:bool)
        n1028 = case shown="False" w688 {
          frame False {
            n1029 = stacked-sequence {
              frame #0 {
                n1030 = Wait (ms)(milliseconds to wait=u32 100) -> ()  [unwired: 1 out]
                n1031 = local write "Slide 25"(u8 100 ("Horizontal Progress Bar 2")) -> ()
              }
              frame #1 {
                n1032 = local write "Slide 25"(u8 90 ("Horizontal Progress Bar 2")) -> ()
                n1033 = Wait (ms)(milliseconds to wait=u32 100) -> ()  [unwired: 1 out]
              }
              frame #2 {
                n1034 = Wait (ms)(milliseconds to wait=u32 100) -> ()  [unwired: 1 out]
                n1035 = local write "Slide 25"(u8 80 ("Horizontal Progress Bar 2")) -> ()
              }
              frame #3 {
                n1036 = local write "Slide 25"(u8 70 ("Horizontal Progress Bar 2")) -> ()
                n1037 = Wait (ms)(milliseconds to wait=u32 100) -> ()  [unwired: 1 out]
              }
              frame #4 {
                n1038 = local write "Slide 25"(u8 60 ("Horizontal Progress Bar 2")) -> ()
                n1039 = Wait (ms)(milliseconds to wait=u32 100) -> ()  [unwired: 1 out]
              }
              frame #5 {
                n1040 = local write "Slide 25"(u8 50 ("Horizontal Progress Bar 2")) -> ()
                n1041 = Wait (ms)(milliseconds to wait=u32 100) -> ()  [unwired: 1 out]
              }
              frame #6 {
                n1042 = local write "Slide 25"(u8 40 ("Horizontal Progress Bar 2")) -> ()
                n1043 = Wait (ms)(milliseconds to wait=u32 100) -> ()  [unwired: 1 out]
              }
              frame #7 {
                n1044 = Wait (ms)(milliseconds to wait=u32 100) -> ()  [unwired: 1 out]
                n1045 = local write "Slide 25"(u8 30 ("Horizontal Progress Bar 2")) -> ()
              }
              frame #8 {
                n1046 = local write "Slide 25"(u8 20 ("Horizontal Progress Bar 2")) -> ()
                n1047 = Wait (ms)(milliseconds to wait=u32 100) -> ()  [unwired: 1 out]
              }
              frame #9 {
                n1048 = Wait (ms)(milliseconds to wait=u32 100) -> ()  [unwired: 1 out]
                n1049 = local write "Slide 25"(u8 10 ("Horizontal Progress Bar 2")) -> ()
              }
              frame #10 {
                n1050 = Wait (ms)(milliseconds to wait=u32 100) -> ()  [unwired: 1 out]
                n1051 = local write "Slide 25"(u8 0 ("Horizontal Progress Bar 2")) -> ()
              }
            }
          }
          frame True {
            n1052 = for {
              N: 55 -> [_]
              i -> [w717]
              stop <- w714 stop-if-true
              n1053 = Multiply(x=w717, y=2) -> (x*y=w712:i32)
              "Slide 25" <- w712
              n1054 = Equal?(x=w712, y=99) -> (x = y?=w714:bool)
              n1055 = Wait (ms)(milliseconds to wait=u32 50) -> ()  [unwired: 1 out]
            }
          }
        }
      }
      frame "60" {
        n1056 = Decimal String To Number(string=w719) -> (number=w718:i32)  [unwired: 2 in, 1 out]
        n1057 = local write "DiningRoom Temprature"(w718) -> ()
      }
      frame "61" {
        n1058 = Decimal String To Number(string=w721) -> (number=w720:i32)  [unwired: 2 in, 1 out]
        n1059 = local write "LivingRoom Temprature"(w720) -> ()
      }
      frame "62" {
        n1060 = Decimal String To Number(string=w723) -> (number=w722:i32)  [unwired: 2 in, 1 out]
        n1061 = local write "Bedroom Temprature"(w722) -> ()
      }
      frame "63" {
        n1062 = Decimal String To Number(string=w725) -> (number=w724:i32)  [unwired: 2 in, 1 out]
        n1063 = local write "MasterRoom Temprature"(w724) -> ()
      }
      frame "64" {
        n1064 = Decimal String To Number(string=w727) -> (number=w726:i32)  [unwired: 2 in, 1 out]
        n1065 = local write "Bedroom2 Temprature"(w726) -> ()
      }
      frame "65" {
        n1066 = Decimal String To Number(string=w729) -> (number=w728:i32)  [unwired: 2 in, 1 out]
        n1067 = local write "LivingRoom2 Temprature"(w728) -> ()
      }
      frame "66" {
        n1068 = Type Cast(type=TRUE, x=w731) -> (*(type *) &x=w730:bool)
        n1069 = local write "Boolean 47"(w730) -> ()
      }
      frame "67" {
        n1070 = Type Cast(type=TRUE, x=w734) -> (*(type *) &x=w733:bool)
        n1071 = local write "Boolean 46"(w733) -> ()
      }
      frame "68" {
        n1072 = Type Cast(type=TRUE, x=w737) -> (*(type *) &x=w736:bool)
        n1073 = local write "Boolean 45"(w736) -> ()
      }
      frame "69" {
        n1074 = Type Cast(type=TRUE, x=w740) -> (*(type *) &x=w739:bool)
        n1075 = local write "Boolean 50"(w739) -> ()
      }
      frame "70" {
        n1076 = Type Cast(type=TRUE, x=w743) -> (*(type *) &x=w742:bool)
        n1077 = local write "Boolean 49"(w742) -> ()
      }
      frame "71" {
        n1078 = Type Cast(type=TRUE, x=w746) -> (*(type *) &x=w745:bool)
        n1079 = local write "Boolean 48"(w745) -> ()
      }
    }
  }
  n1080 = property on="WindowsMediaPlayer 2" class="AXCont"("Visible"=FALSE) -> ()  [unwired: 2 in, 2 out]
  n1081 = while {
    stop <- "stop 3" stop-if-true
    n1082 = flat-sequence {
      frame #0 {
        w749 = TRUE ("Boolean 51")
        n1083 = Wait (ms)(milliseconds to wait=u32 500) -> ()  [unwired: 1 out]
        "Boolean 51" <- w749
        "Boolean 53" <- w749
        "Boolean 54" <- w749
        "Boolean 52" <- w749
      }
      frame #1 {
        w751 = FALSE ("Boolean 51")
        n1084 = local write "Boolean 51"(w751) -> ()
        n1085 = local write "Boolean 54"(w751) -> ()
        n1086 = local write "Boolean 52"(w751) -> ()
        n1087 = Wait (ms)(milliseconds to wait=u32 500) -> ()  [unwired: 1 out]
        n1088 = local write "Boolean 53"(w751) -> ()
      }
    }
  }
  n1089 = while {
    stop <- "stop 2" stop-if-true
    n1090 = property on="WindowsMediaPlayer" class="AXCont"("Height"=u32 289 ("Container Bounds:Height"), "Width"=u32 441 ("Container Bounds:Width")) -> ()  [unwired: 2 in, 2 out]
  }
  n1091 = TCP Close Connection(connection ID=w7, error in (no error)=w5) -> (error out=w2:errorcluster)  [unwired: 1 in, 1 out]
  n1092 = call <vilib>:"Clear Errors.vi"("error in (no error)"=w2) -> ()  [unwired: 6 in, 1 out]
